vi "Phi Theta Scanning Revamped.vi"() -> ()   [LabVIEW 2022 SP3]
uses:
  C:/Users/mnopl/OneDrive/Documents/PhiThetaScanning/Thorlabs.MotionControl.Controls.dll
  Thorlabs.MotionControl.Controls.dll
  <vilib>/DAQmx/read.llb/DAQmx Read (Analog 1D DBL 1Chan NSamp).vi
  <vilib>/Analysis/baseanly.llb/Mean (DBL).vi
  <vilib>/DAQmx/miscellaneous.llb/DAQmx Fill In Error Info.vi
  C:/Users/mnopl/OneDrive/Documents/PhiThetaScanning/Thorlabs.MotionControl.KCube.StepperMotorCLI.dll
  Thorlabs.MotionControl.KCube.StepperMotorCLI.dll
  <vilib>/Analysis/NI_AALBase.lvlib
panel:
  in  "2D Flyover":bool
  in  "Flyover Y Linescan":bool
  in  "Update Vel/Acc":bool
  in  "Save Line graph":bool
  in  "Grid points":dbl=3000.0
  in  "Save Phi/Theta":bool
  out "Time Left":dbl
  out "Line Scan":dbl[](graph)
  in  "Move to Saved Pos":bool
  in  "Save Position":bool
  out "Y Pos 1":dbl
  out "X Pos 1":dbl
  out "return value":dbl[][](array[numeric])
  in  "Save Data":bool
  in  "Move to Origin":bool
  in  "Acceleration":dbl=10.0
  in  "Mesuares/Pixel":dbl=100.0
  in  "Flyover X Linescan":bool
  in  "Move Y":bool
  in  "Move X":bool
  in  "Y Step Size":dbl=1.0
  in  "X Step Size":dbl=1.0
  in  "Move to Y":bool
  in  "Move to X":bool
  in  "Y Move":dbl=1.0
  in  "X Move":dbl=1.0
  out "Y Line Scan":dbl[](array[numeric])=[-inf, -inf, -inf, -inf, -inf, -inf]
  out "X Line Scan":dbl[](array[numeric])=[-inf, -inf, -inf, -inf, -inf, -inf]
  out "Y Origin":dbl
  out "X Orign":dbl
  out "Scan Type":string="Scan"
  in  "Y Line Scan":bool
  in  "Abort":bool
  in  "X Line Scan":bool
  out "(X,Y)":cluster{dbl, dbl}[][](array[cluster])
  out "Phi Theta Data":dbl[][](graph)
  in  "Save Image":bool
  in  "Convert to phi/theta":bool
  in  "Move to Cursor":bool
  in  "Y Pos":dbl=0.899996795693412
  in  "X Pos":dbl=1.0
  in  "Read Position":bool
  out "Graph":dbl[][](graph)
  out "array of values":dbl[][](array[numeric])=[[-inf, -inf, -inf, -inf, -inf, -inf], [-inf, -inf, -inf, -inf, -inf, -inf], [-inf, -inf, -inf, -inf, -inf, -inf], [-inf, -inf, -inf, -inf, -inf, -inf], [-inf, -inf, -inf, -inf, -inf, -inf], [-inf, -inf, -inf, -inf, -inf, -inf]]
  out "task out":refnum<k21>
  in  "physical channels":tag="Dev3/ai0"
  in  "number of samples":i32=10000
  in  "rate":dbl=250000.0
  in  "maximum value":dbl=5.0 format="%0.2f"
  in  "minimum value":dbl=-5.0 format="%0.2f"
  in  "Take Single Measurement":bool
  out "Done Mov?":bool=TRUE
  in  "Y Length":dbl=5.0
  in  "X Length":dbl=5.0
  in  "2D Scan":bool
  in  "Velocity":dbl=2.0
  in  "Move Y (in)":bool
  in  "Move X (in)":bool
  in  "Time to wait":dbl=251.0
  out "Time":i32=77055304
  in  "Y Step Size (in)":dbl=1.0
  in  "X Step Size (in)":dbl=1.0
  in  "X=T,Y=F":bool
  in  "Moving?":bool
  in  "Stop":bool
  in  "KCubeStepperControl Y":refnum<k24>(container)
  in  "KCubeStepperControl X":refnum<k24>(container)
  in  "SerialNumber X":string="26005327"
  in  "SerialNumber Y":string="26005279"
  in  "Set Vel/Acc":bool
  # "Internal Variables"
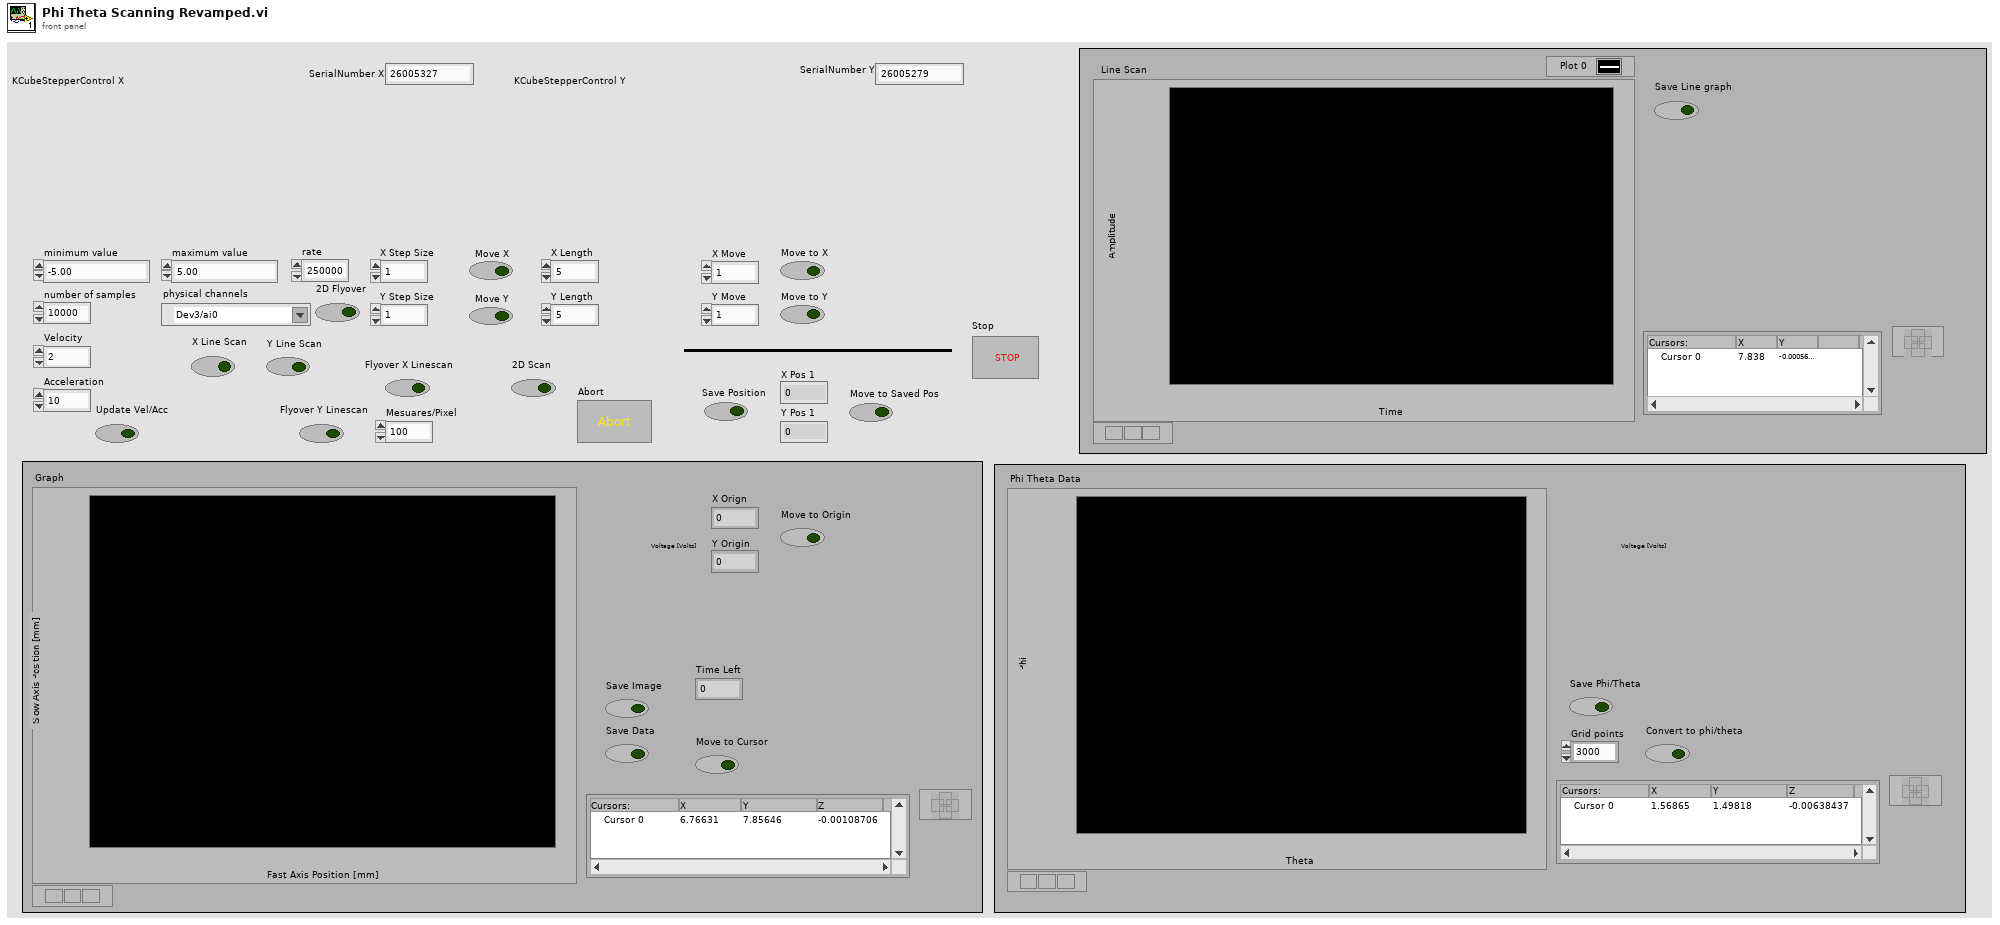
[diagram p1: front panel]
types:
  T1 = typedef "LVPointDoubleTypeDef.ctl" = cluster{"Cursor X":dbl, "Cursor Y":dbl}
  T2 = typedef "imagedata.ctl" = cluster{"image type":i32, "image depth":i32, "image":u8[], "mask":u8[], "colors":u32[], "Rectangle":cluster{"left":i16, "top":i16, "right":i16, "bottom":i16}}
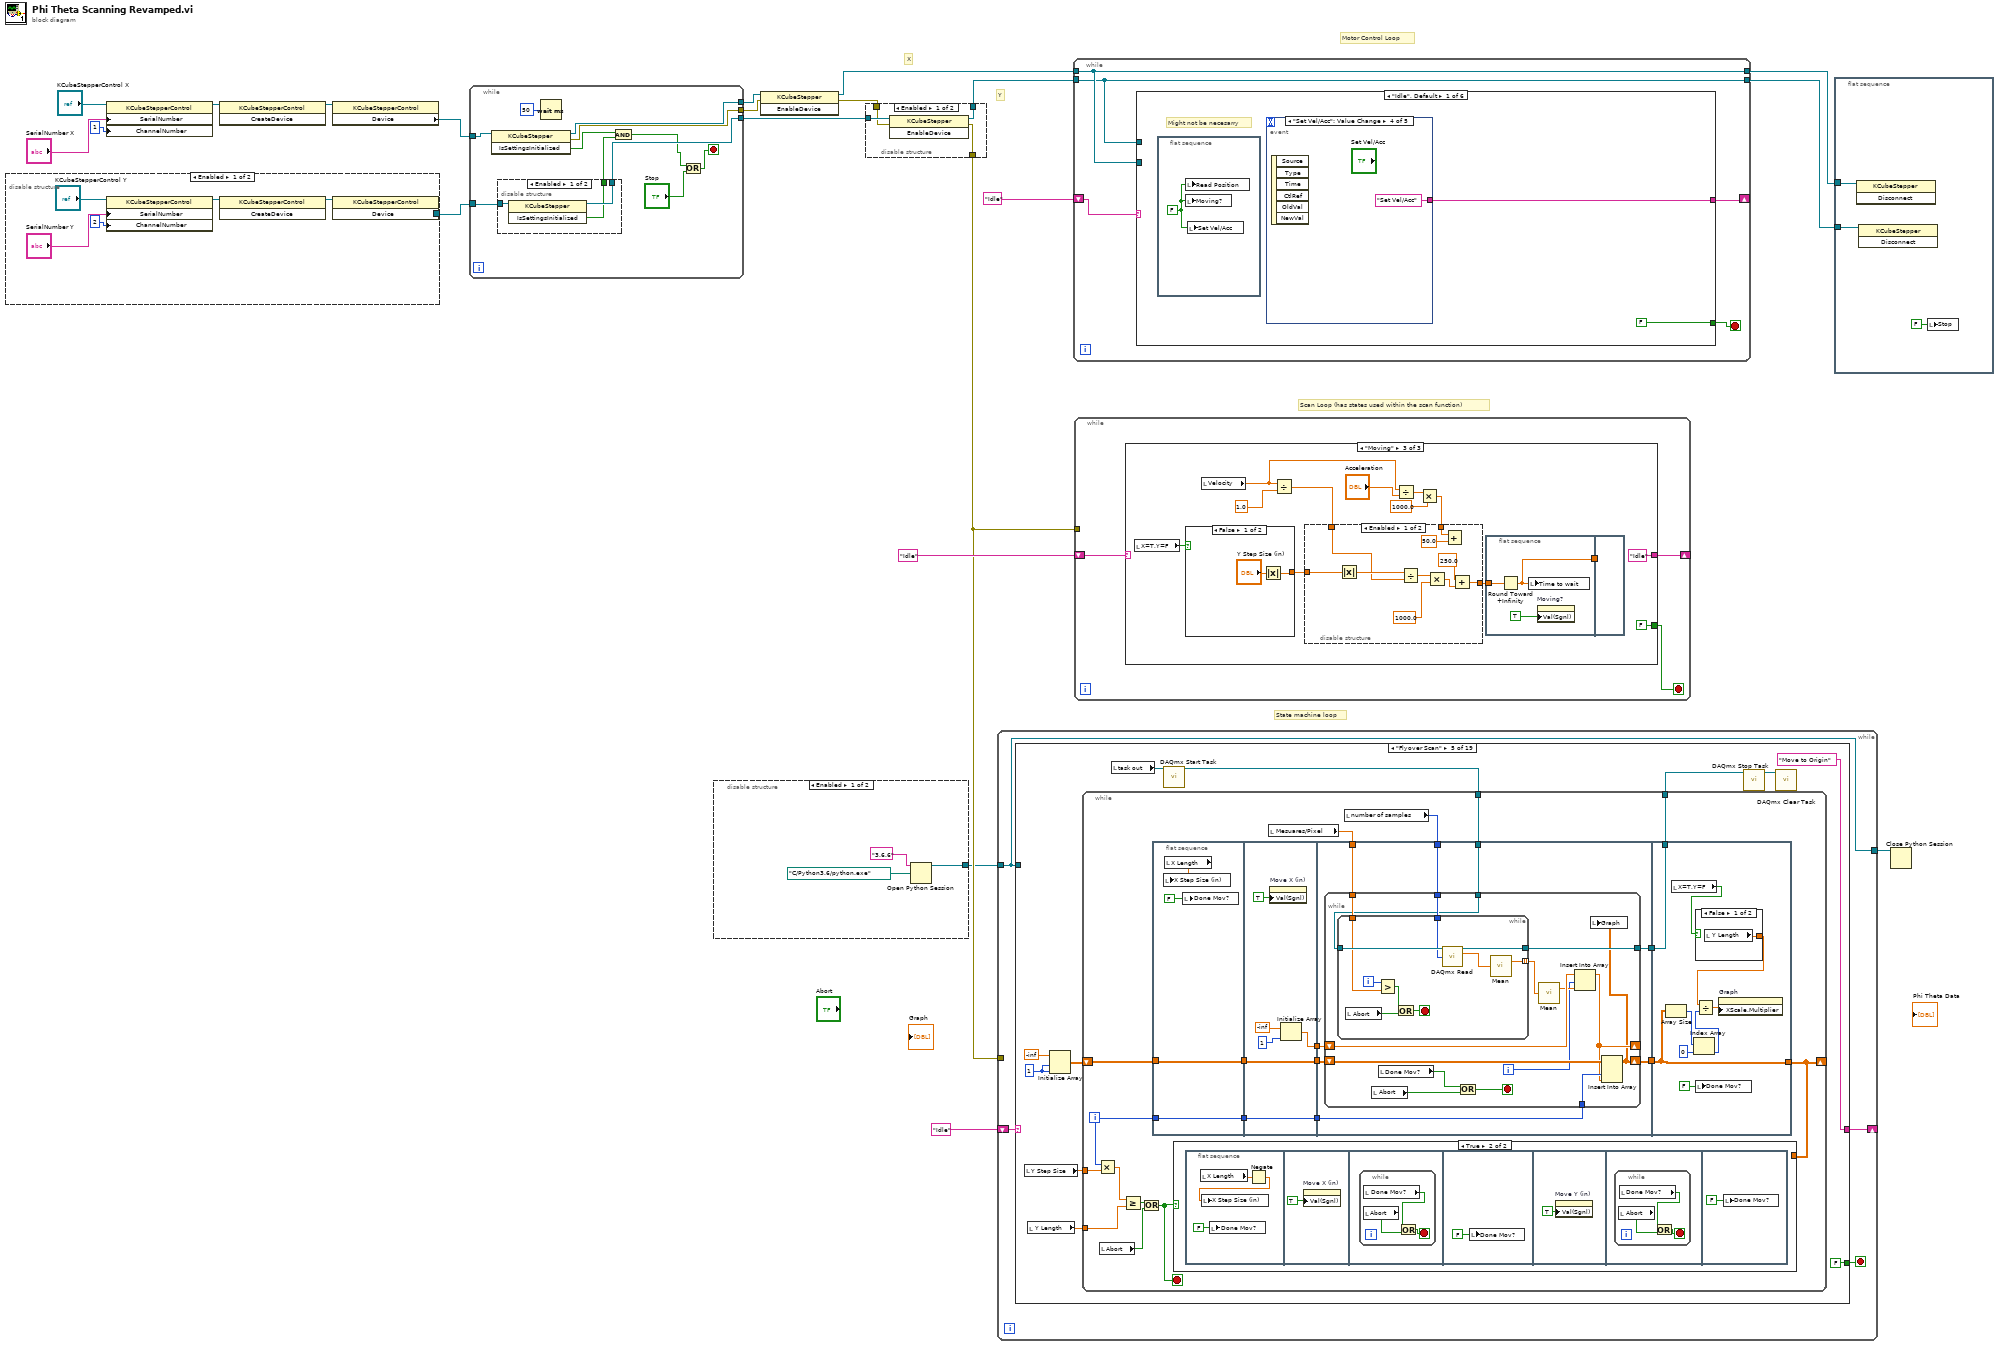
[diagram p0: block diagram]
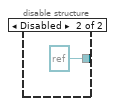
[diagram p2: hidden frame]
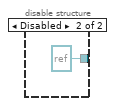
[diagram p4: hidden frame]
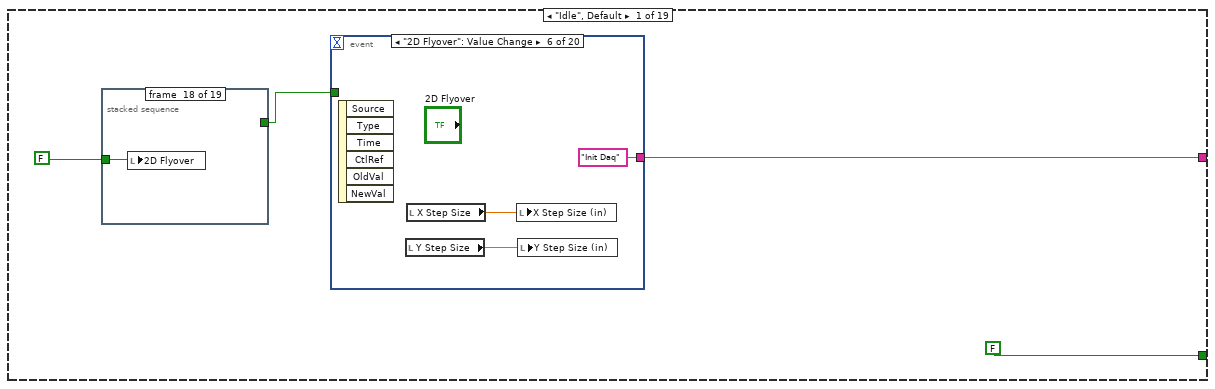
[diagram p5: hidden frame]
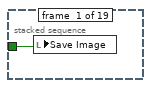
[diagram p6: hidden frame]
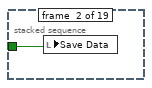
[diagram p7: hidden frame]
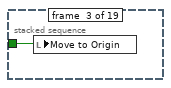
[diagram p8: hidden frame]
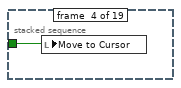
[diagram p9: hidden frame]
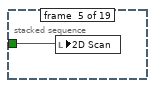
[diagram p10: hidden frame]
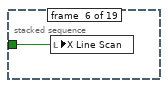
[diagram p11: hidden frame]
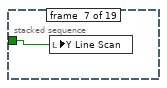
[diagram p12: hidden frame]
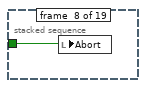
[diagram p13: hidden frame]
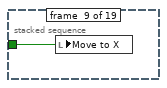
[diagram p14: hidden frame]
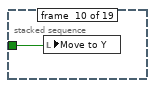
[diagram p15: hidden frame]
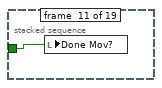
[diagram p16: hidden frame]
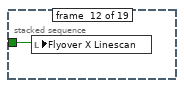
[diagram p17: hidden frame]
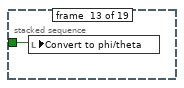
[diagram p18: hidden frame]
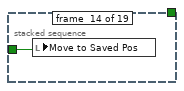
[diagram p19: hidden frame]
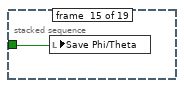
[diagram p20: hidden frame]
diagram:
  # "State machine loop"
  # "Y"
  # "X"
  # "Scan Loop (has states used within the scan function)"
  # "Motor Control Loop"
  n1 = disable-structure shown="Enabled" {
    disable-tunnel: [w23 refnum<k24> refnum ("Device")] -> w13
    frame Enabled {
      n2 = property class="KCubeStepperControl"(reference="KCubeStepperControl Y", "SerialNumber"="SerialNumber Y", "ChannelNumber"=2) -> (reference out=w26:refnum<k24>)  [unwired: 1 in, 1 out]
      n3 = invoke class="KCubeStepperControl" method="CreateDevice"(reference=w26) -> (reference out=w25:refnum<k24>)  [unwired: 2 in, 2 out]
      n4 = property class="KCubeStepperControl"(reference=w25) -> ("Device"=w23:refnum<k24>)  [unwired: 1 in, 2 out]
    }
    frame Disabled {
    }
  }
  n5 = property class="KCubeStepperControl"(reference="KCubeStepperControl X", "SerialNumber"="SerialNumber X", "ChannelNumber"=1) -> (reference out=w20:refnum<k24>)  [unwired: 1 in, 1 out]
  n6 = invoke class="KCubeStepperControl" method="CreateDevice"(reference=w20) -> (reference out=w19:refnum<k24>)  [unwired: 2 in, 2 out]
  n7 = property class="KCubeStepperControl"(reference=w19) -> ("Device"=w18:refnum<k24>)  [unwired: 1 in, 2 out]
  n8 = while {
    tunnel: w13 -> [w38]
    tunnel: w18 -> [w32]
    tunnel: [w35] -> w17
    tunnel: [w36] -> w15
    tunnel: [w37] -> w14
    stop <- w31 stop-if-true
    n9 = invoke class="KCubeStepper" method="IsSettingsInitialized"(reference=w32) -> (reference out=w36:refnum<k24>, error out=w37:errorcluster, "IsSettingsInitialized"=w33:bool)  [unwired: 2 in]
    n10 = disable-structure shown="Enabled" {
      disable-tunnel: w38 -> [w42 w43]
      disable-tunnel: [w41 w43] -> w35
      disable-tunnel: [w40 TRUE ("IsSettingsInitialized")] -> w34
      frame Enabled {
        n11 = invoke class="KCubeStepper" method="IsSettingsInitialized"(reference=w42) -> (reference out=w41:refnum<k24>, "IsSettingsInitialized"=w40:bool)  [unwired: 2 in, 1 out]
      }
      frame Disabled {
      }
    }
    n12 = Wait (ms)(milliseconds to wait=u32 50) -> ()  [unwired: 1 out]
    n13 = And(x=w33, y=w34) -> (x .and. y?=w29:bool)
    n14 = Or(x=w29, y="Stop") -> (x .or. y?=w31:bool)
  }
  n15 = disable-structure shown="Enabled" {
    disable-tunnel: [w47 refnum<k35> refnum ("session out")] -> w4
    frame Enabled {
      n16 = Open Python Session(python version="3.6.6" ("Python version"), python path=path "C:/Python3.6/python.exe" ("Python path")) -> (session out=w47:refnum<k35>)  [unwired: 1 in, 1 out]
    }
    frame Disabled {
    }
  }
  n17 = invoke class="KCubeStepper" method="EnableDevice"(reference=w15, error in=w14) -> (reference out=w2:refnum<k24>, error out=w12:errorcluster)  [unwired: 1 in, 1 out]
  n18 = disable-structure shown="Enabled" {
    disable-tunnel: w17 -> [w52 _]
    disable-tunnel: w12 -> [w51 w53]
    disable-tunnel: [w50 w53] -> w5
    disable-tunnel: [w49 _] -> w1
    frame Enabled {
      n19 = invoke class="KCubeStepper" method="EnableDevice"(reference=w52, error in=w51) -> (reference out=w49:refnum<k24>, error out=w50:errorcluster)  [unwired: 1 in, 1 out]
    }
    frame Disabled {
    }
  }
  n20 = while {
    shift-right: [w56] -> _
    shift-left: "Idle" -> [w57]
    tunnel: w5 -> [_]
    tunnel: w4 -> [w54]
    tunnel: [w54] -> w3
    stop <- w55 stop-if-true
    n21 = case shown="\"Flyover Scan\"" w57 {
      tunnel: [w61 "Init Graph" w152 "Move to Origin" "Move to Origin" ("Scan Type") "Move to Origin" ("Scan Type") "Move to Origin" ("Scan Type") "Idle" ("Scan Type") "Idle" ("Scan Type") "Idle" "Idle" ("Scan Type") "Idle" ("Scan Type") "Idle" "Idle" ("Scan Type") "Idle" "Idle" ("Scan Type") "Idle" ("Scan Type") "Idle" ("Scan Type") "Idle"] -> w56
      tunnel: [FALSE FALSE FALSE FALSE FALSE FALSE FALSE FALSE FALSE FALSE FALSE FALSE FALSE FALSE FALSE FALSE FALSE FALSE TRUE] -> w55
      tunnel: w54 -> [_ _ _ _ _ _ _ _ _ _ _ _ w791 _ _ w928 _ _ _]
      frame "Idle", Default {
        n22 = stacked-sequence {
          tunnel: FALSE -> [w62 w63 w64 w65 w66 w67 w68 w69 w70 w71 w72 w73 w74 w75 w76 w77 w78 w79 w80]
          tunnel: [_ _ _ _ _ _ _ _ _ _ _ _ _ _ _ _ _ _ w80] -> w58
          frame #0 {
            n23 = local write "Save Image"(w62) -> ()
          }
          frame #1 {
            n24 = local write "Save Data"(w63) -> ()
          }
          frame #2 {
            n25 = local write "Move to Origin"(w64) -> ()
          }
          frame #3 {
            n26 = local write "Move to Cursor"(w65) -> ()
          }
          frame #4 {
            n27 = local write "2D Scan"(w66) -> ()
          }
          frame #5 {
            n28 = local write "X Line Scan"(w67) -> ()
          }
          frame #6 {
            n29 = local write "Y Line Scan"(w68) -> ()
          }
          frame #7 {
            n30 = local write "Abort"(w69) -> ()
          }
          frame #8 {
            n31 = local write "Move to X"(w70) -> ()
          }
          frame #9 {
            n32 = local write "Move to Y"(w71) -> ()
          }
          frame #10 {
            n33 = local write "Done Mov?"(w72) -> ()
          }
          frame #11 {
            n34 = local write "Flyover X Linescan"(w73) -> ()
          }
          frame #12 {
            n35 = local write "Convert to phi/theta"(w74) -> ()
          }
          frame #13 {
            n36 = local write "Move to Saved Pos"(w75) -> ()
          }
          frame #14 {
            n37 = local write "Save Phi/Theta"(w76) -> ()
          }
          frame #15 {
            n38 = local write "Update Vel/Acc"(w77) -> ()
          }
          frame #16 {
            n39 = local write "Flyover Y Linescan"(w78) -> ()
          }
          frame #17 {
            n40 = local write "2D Flyover"(w79) -> ()
          }
          frame #18 {
            n41 = local write "Save Position"(w80) -> ()
          }
        }
        n42 = event shown="[5] \"2D Flyover\": Value Change" {
          selector: _ -> [_ _ _ _ _ _ _ _ _ _ _ _ _ _ _ _ _ _ _ _]
          dyn-events: _ -> [_ _ _ _ _ _ _ _ _ _ _ _ _ _ _ _ _ _ _ _]
          timeout: _ -> [_ _ _ _ _ _ _ _ _ _ _ _ _ _ _ _ _ _ _ _]
          tunnel: ["Idle" "Convert" "Move to Cursor" "Stop" "Init Daq" "Init Daq" "Move to Origin" "Move to Saved Position" "Init Daq" "Init Daq" "Init Daq" "Init Daq" "Move to" "Move to" "Update Vel/Acc" "Save Position" "Save Image" "Save Phi/Theta" "Save Line graph" "Save Data"] -> w61
          tunnel: w58 -> [_ _ _ _ _ _ _ _ _ _ _ _ _ _ _ _ _ _ _ _]
          event Timeout {
            n43 = event-data() -> ()  [unwired: 1 in, 3 out]
          }
          event "Convert to phi/theta": Value Change {
            n44 = event-data() -> ()  [unwired: 1 in, 6 out]
          }
          event "Move to Cursor": Value Change {
            n45 = event-data() -> ()  [unwired: 1 in, 6 out]
          }
          event "Stop": Value Change {
            n46 = event-data() -> ()  [unwired: 1 in, 6 out]
          }
          event "2D Scan": Value Change {
            n47 = event-data() -> ()  [unwired: 1 in, 6 out]
            n48 = local read "X Step Size"() -> (w85:dbl)
            n49 = local read "Y Step Size"() -> (w86:dbl)
            n50 = local write "Scan Type"("Scan" ("Scan Type")) -> ()
            n51 = local write "Y Step Size (in)"(w86) -> ()
            n52 = local write "X Step Size (in)"(w85) -> ()
          }
          event "2D Flyover": Value Change {
            n53 = event-data() -> ()  [unwired: 1 in, 6 out]
            n54 = local read "Y Step Size"() -> (w89:dbl)
            n55 = local read "X Step Size"() -> (w90:dbl)
            n56 = local write "X Step Size (in)"(w90) -> ()
            n57 = local write "Y Step Size (in)"(w89) -> ()
          }
          event "Move to Origin": Value Change {
            n58 = event-data() -> ()  [unwired: 1 in, 6 out]
          }
          event "Move to Saved Pos": Value Change {
            n59 = event-data() -> ()  [unwired: 1 in, 6 out]
          }
          event "X Line Scan": Value Change {
            n60 = event-data() -> ()  [unwired: 1 in, 6 out]
            n61 = local read "X Step Size"() -> (w94:dbl)
            n62 = local write "X Step Size (in)"(w94) -> ()
            n63 = local write "Scan Type"("Line Scan" ("Scan Type")) -> ()
            n64 = local write "X=T,Y=F"(TRUE ("X=T,Y=F")) -> ()
          }
          event "Flyover X Linescan": Value Change {
            n65 = event-data() -> ()  [unwired: 1 in, 6 out]
            n66 = local read "X Step Size"() -> (w101:dbl)
            n67 = local write "X Step Size (in)"(w101) -> ()
            n68 = local write "Scan Type"("Flyover Linescan" ("Scan Type")) -> ()
            n69 = local write "X=T,Y=F"(TRUE ("X=T,Y=F")) -> ()
          }
          event "Flyover Y Linescan": Value Change {
            n70 = event-data() -> ()  [unwired: 1 in, 6 out]
            n71 = local read "Y Step Size"() -> (w103:dbl)
            n72 = local write "Y Step Size (in)"(w103) -> ()
            n73 = local write "Scan Type"("Flyover Linescan" ("Scan Type")) -> ()
            n74 = local write "X=T,Y=F"(FALSE ("X=T,Y=F")) -> ()
          }
          event "Y Line Scan": Value Change {
            n75 = event-data() -> ()  [unwired: 1 in, 6 out]
            n76 = local read "Y Step Size"() -> (w106:dbl)
            n77 = local write "Y Step Size (in)"(w106) -> ()
            n78 = local write "X=T,Y=F"(FALSE ("X=T,Y=F")) -> ()
            "Scan Type" <- "Line Scan" ("Scan Type")
          }
          event "Move to X": Value Change {
            n79 = event-data() -> ()  [unwired: 1 in, 6 out]
            n80 = local write "X=T,Y=F"(TRUE ("X=T,Y=F")) -> ()
          }
          event "Move to Y": Value Change {
            n81 = event-data() -> ()  [unwired: 1 in, 6 out]
            n82 = local write "X=T,Y=F"(FALSE ("X=T,Y=F")) -> ()
          }
          event "Update Vel/Acc": Value Change {
            n83 = event-data() -> ()  [unwired: 1 in, 6 out]
          }
          event "Save Position": Value Change {
            n84 = event-data() -> ()  [unwired: 1 in, 6 out]
          }
          event "Save Image": Value Change {
            n85 = event-data() -> ()  [unwired: 1 in, 6 out]
          }
          event "Save Phi/Theta": Value Change {
            n86 = event-data() -> ()  [unwired: 1 in, 6 out]
          }
          event "Save Line graph": Value Change {
            n87 = event-data() -> ()  [unwired: 1 in, 6 out]
          }
          event "Save Data": Value Change {
            n88 = event-data() -> ()  [unwired: 1 in, 6 out]
          }
        }
      }
      frame "Init Daq" {
        w120 = -inf
        n89 = local read "Y Length"() -> (w133:dbl)
        n90 = local read "Y Step Size"() -> (w132:dbl)
        n91 = local read "X Length"() -> (w130:dbl)
        n92 = local read "X Step Size"() -> (w129:dbl)
        n93 = Divide(x=w133, y=w132) -> (x/y=w134:dbl)
        n94 = Divide(x=w130, y=w129) -> (x/y=w131:dbl)
        n95 = Round Toward +Infinity(x=w134) -> (ceil(x): smallest int >= x=w123:dbl)
        n96 = Round Toward +Infinity(x=w131) -> (ceil(x): smallest int >= x=w128:dbl)
        n97 = Increment(x=w123) -> (x+1=w121:dbl)
        n98 = Increment(x=w128) -> (x+1=w122:dbl)
        n99 = call "Initialize DAQ Assistant.vi"("minimum value"="minimum value", "maximum value"="maximum value", "rate"="rate", "number of samples"="number of samples", "physical channels"="physical channels") -> ("task out"=→"task out":refnum<k21>)  [unwired: 5 in, 1 out]
        n100 = Initialize Array(w120, w121) -> (→"Y Line Scan":dbl[])
        n101 = Initialize Array(w120, w122, w121) -> (→"array of values":dbl[][])
        n102 = Initialize Array(w120, w122) -> (→"X Line Scan":dbl[])
      }
      frame "Init Graph" {
        n103 = local read "Acceleration"() -> (w148:dbl)
        n104 = local read "Scan Type"() -> (w152:string)
        n105 = local read "Velocity"() -> (w149:dbl)
        n106 = flat-sequence {
          tunnel: [w205] -> w142
          tunnel: ["X Pos"] -> w154
          tunnel: ["Y Pos"] -> w153
          frame #0 {
            n107 = property on="Read Position" class="Bool (strict)"("Val(Sgnl)"=TRUE) -> ()  [unwired: 2 in, 2 out]
          }
          frame #1 {
            n108 = while {
              tunnel: [w206] -> w205
              stop <- w209 stop-if-true
              n109 = local read "Read Position"() -> (w208:bool)
              n110 = Not(x=w208) -> (.not. x?=w209:bool)
              n111 = Wait (ms)(milliseconds to wait=u32 10) -> (millisecond timer value=w206:u32)
            }
          }
          frame #2 {
            "X Orign" <- "X Pos"
            "Y Origin" <- "Y Pos"
          }
        }
        n112 = case shown="\"Scan\"" w152 {
          tunnel: [w170 w188] -> w146
          tunnel: w145 -> [w170 w188]
          frame "Line Scan", Default {
            n113 = local read "X=T,Y=F"() -> (w171:bool)
            n114 = case shown="True" w171 {
              frame False {
                n115 = flat-sequence {
                  frame #0 {
                    n116 = local read "Y Length"() -> (w173:dbl)
                    n117 = Divide(x=w173, y=2.0) -> (x/y=w174:dbl)
                    n118 = Negate(x=w174) -> (-x=w175:dbl)
                    n119 = local write "Y Step Size (in)"(w175) -> ()
                  }
                  frame #1 {
                    n120 = local write "Done Mov?"(FALSE ("Done Mov?")) -> ()
                    n121 = property on="Move Y (in)" class="Bool (strict)"("Val(Sgnl)"=TRUE ("Value (Signaling)")) -> ()  [unwired: 2 in, 2 out]
                  }
                  frame #2 {
                    n122 = while {
                      stop <- w178 stop-if-true
                      n123 = local read "Done Mov?"() -> (w178:bool)
                    }
                  }
                  frame #3 {
                    n124 = local write "Done Mov?"(FALSE ("Done Mov?")) -> ()
                  }
                }
              }
              frame True {
                n125 = flat-sequence {
                  frame #0 {
                    n126 = local read "X Length"() -> (w183:dbl)
                    n127 = Divide(x=w183, y=2.0) -> (x/y=w182:dbl)
                    n128 = Negate(x=w182) -> (-x=w181:dbl)
                    n129 = local write "X Step Size (in)"(w181) -> ()
                  }
                  frame #1 {
                    n130 = property on="Move X (in)" class="Bool (strict)"("Val(Sgnl)"=TRUE ("Value (Signaling)")) -> ()  [unwired: 2 in, 2 out]
                    n131 = local write "Done Mov?"(FALSE ("Done Mov?")) -> ()
                  }
                  frame #2 {
                    n132 = while {
                      stop <- w186 stop-if-true
                      n133 = local read "Done Mov?"() -> (w186:bool)
                    }
                  }
                  frame #3 {
                    n134 = local write "Done Mov?"(FALSE ("Done Mov?")) -> ()
                  }
                }
              }
            }
          }
          frame "Scan" {
            n135 = flat-sequence {
              frame #0 {
                n136 = local read "X Length"() -> (w196:dbl)
                n137 = local read "Y Length"() -> (w194:dbl)
                n138 = Divide(x=w196, y=2.0) -> (x/y=w192:dbl)
                n139 = Divide(x=w194, y=2.0) -> (x/y=w190:dbl)
                n140 = Negate(x=w192) -> (-x=w191:dbl)
                n141 = Negate(x=w190) -> (-x=w189:dbl)
                n142 = local write "X Step Size (in)"(w191) -> ()
                n143 = local write "Y Step Size (in)"(w189) -> ()
              }
              frame #1 {
                n144 = local write "Done Mov?"(FALSE ("Done Mov?")) -> ()
                n145 = property on="Move Y (in)" class="Bool (strict)"("Val(Sgnl)"=TRUE ("Value (Signaling)")) -> ()  [unwired: 2 in, 2 out]
              }
              frame #2 {
                n146 = while {
                  stop <- w199 stop-if-true
                  n147 = local read "Done Mov?"() -> (w199:bool)
                }
              }
              frame #3 {
                n148 = local write "Done Mov?"(FALSE ("Done Mov?")) -> ()
                n149 = property on="Move X (in)" class="Bool (strict)"("Val(Sgnl)"=TRUE ("Value (Signaling)")) -> ()  [unwired: 2 in, 2 out]
              }
              frame #4 {
                n150 = while {
                  stop <- w202 stop-if-true
                  n151 = local read "Done Mov?"() -> (w202:bool)
                }
              }
              frame #5 {
                n152 = local write "Done Mov?"(FALSE ("Done Mov?")) -> ()
              }
            }
          }
        }
        n153 = flat-sequence {
          tunnel: w149 -> [w159]
          tunnel: [w159] -> w151
          tunnel: w148 -> [w156]
          tunnel: [w156] -> w150
          tunnel: w142 -> [_]
          tunnel: w151 -> [w162]
          tunnel: w150 -> [w161]
          tunnel: [w162] -> w144
          tunnel: [w161] -> w143
          tunnel: [w164] -> w145
          tunnel: [w165] -> w147
          tunnel: w144 -> [w165]
          tunnel: w143 -> [w164]
          frame #0 {
            n154 = local write "Acceleration"(10.0 ("Acceleration")) -> ()
            n155 = local write "Velocity"(2.0 ("Velocity")) -> ()
          }
          frame #1 {
            n156 = property on="Set Vel/Acc" class="Bool (strict)"("Val(Sgnl)"=TRUE ("Value (Signaling)")) -> ()  [unwired: 2 in, 2 out]
          }
          frame #2 {
            n157 = Wait (ms)(milliseconds to wait=u32 150) -> ()  [unwired: 1 out]
          }
        }
        n158 = case shown="\"Scan\"" w152 {
          tunnel: w154 -> [w215 w234]
          tunnel: w153 -> [w214 w229]
          frame "Line Scan", Default {
            n159 = local read "X=T,Y=F"() -> (w213:bool)
            n160 = case shown="False" w213 {
              tunnel: w215 -> [_ w227]
              tunnel: w214 -> [w221 _]
              tunnel: [w216 w222] -> w212
              frame False {
                n161 = local read "Y Length"() -> (w219:dbl)
                n162 = local read "Y Step Size"() -> (w216:dbl)
                n163 = Divide(x=w219, y=2.0) -> (x/y=w217:dbl)
                n164 = Subtract(x=w221, y=w217) -> (x-y=w220:dbl)
                n165 = property on="Line Scan" class="WFGraph (strict)"("XScale.Offset"=w220) -> ()  [unwired: 2 in, 2 out]
              }
              frame True {
                n166 = local read "X Length"() -> (w225:dbl)
                n167 = Divide(x=w225, y=2.0) -> (x/y=w223:dbl)
                n168 = Subtract(x=w227, y=w223) -> (x-y=w226:dbl)
                n169 = local read "X Step Size"() -> (w222:dbl)
                n170 = property on="Line Scan" class="WFGraph (strict)"("XScale.Offset"=w226) -> ()  [unwired: 2 in, 2 out]
              }
            }
            n171 = property on="Line Scan" class="WFGraph (strict)"("XScale.Multiplier"=w212) -> ()  [unwired: 2 in, 2 out]
          }
          frame "Scan" {
            n172 = local read "X Length"() -> (w237:dbl)
            n173 = local read "Y Length"() -> (w232:dbl)
            n174 = Divide(x=w237, y=2.0) -> (x/y=w235:dbl)
            n175 = Divide(x=w232, y=2.0) -> (x/y=w230:dbl)
            n176 = local read "Y Step Size"() -> (w239:dbl)
            n177 = local read "X Step Size"() -> (w238:dbl)
            n178 = Subtract(x=w229, y=w230) -> (x-y=w228:dbl)
            n179 = Subtract(x=w234, y=w235) -> (x-y=w233:dbl)
            n180 = property on="Graph" class="IntGraph (strict)"("XScale.Offset"=w233) -> ()  [unwired: 2 in, 2 out]
            n181 = property on="Graph" class="IntGraph (strict)"("YScale.Offset"=w228) -> ()  [unwired: 2 in, 2 out]
            n182 = property on="Graph" class="IntGraph (strict)"("YScale.Multiplier"=w239) -> ()  [unwired: 2 in, 2 out]
            n183 = property on="Graph" class="IntGraph (strict)"("XScale.Multiplier"=w238) -> ()  [unwired: 2 in, 2 out]
          }
        }
        n184 = flat-sequence {
          tunnel: w146 -> [w167]
          tunnel: w147 -> [w166]
          frame #0 {
            n185 = local write "Velocity"(w166) -> ()
            n186 = local write "Acceleration"(w167) -> ()
          }
          frame #1 {
            n187 = property on="Set Vel/Acc" class="Bool (strict)"("Val(Sgnl)"=TRUE ("Value (Signaling)")) -> ()  [unwired: 2 in, 2 out]
          }
          frame #2 {
            n188 = Wait (ms)(milliseconds to wait=u32 150) -> ()  [unwired: 1 out]
          }
        }
      }
      frame "Scan" {
        w248 = 0 ("Row")
        n189 = local read "number of samples"() -> (w244:i32)
        n190 = local read "Y Step Size"() -> (w242:dbl)
        n191 = local read "array of values"() -> (w246:dbl[][])
        n192 = local read "Y Origin"() -> (w253:dbl)
        n193 = local read "task out"() -> (w247:refnum<k21>)
        n194 = local read "X Orign"() -> (w255:dbl)
        n195 = local read "X Step Size"() -> (w259:dbl)
        n196 = Divide(x="Y Length", y=2.0) -> (x/y=w251:dbl)
        n197 = Divide(x="X Length", y=2.0) -> (x/y=w254:dbl)
        n198 = Divide(x="Y Length", y=w242) -> (x/y=w241:dbl)
        n199 = call "Measure and Update Array.vi"("Array In"=w246, "number of samples per channel"=w244, "task/channels in"=w247, "Row"=w248, "Column"=w248) -> ("Array Out"=w245:dbl[][])  [unwired: 7 in, 3 out]
        n200 = local write "Graph"(w245) -> ()
        n201 = Subtract(x=w253, y=w251) -> (x-y=w249:dbl)
        n202 = Subtract(x=w255, y=w254) -> (x-y=w250:dbl)
        n203 = while {
          shift-right: [w294] -> w261
          shift-left: w245 -> [w295]
          tunnel: [w290] -> w260 mode=indexing
          tunnel: "X Length" -> [w286]
          tunnel: w259 -> [w289]
          tunnel: w242 -> [w288]
          tunnel: "Y Length" -> [w287]
          tunnel: [w280] -> w258
          tunnel: "X Length" -> [w285]
          tunnel: w250 -> [w279]
          tunnel: w249 -> [w278]
          tunnel: w241 -> [w273]
          i -> [w292]
          stop <- w297 stop-if-true
          n204 = local read "Abort"() -> (w281:bool)
          n205 = Multiply(x=w292, y=w288) -> (x*y=w291:dbl)
          n206 = while {
            tunnel: [w404] -> w284
            tunnel: w292 -> [w404]
            tunnel: [w403] -> w296
            shift-right: [w399] -> w283
            shift-left: w295 -> [w402]
            tunnel: [w401] -> w282
            tunnel: [w400] -> w293
            tunnel: w291 -> [w390]
            tunnel: [w398] -> w290 mode=indexing
            tunnel: w286 -> [w396]
            tunnel: w289 -> [w397]
            tunnel: w279 -> [w389]
            tunnel: w278 -> [w387]
            i -> [w411]
            stop <- w408 stop-if-true
            n207 = flat-sequence {
              tunnel: w397 -> [w412]
              tunnel: w396 -> [w413]
              tunnel: w411 -> [w414]
              tunnel: [w414] -> w395
              tunnel: [w413] -> w394
              tunnel: [w412] -> w393
              tunnel: [w422] -> w410
              tunnel: [w416] -> w405
              tunnel: [w421] -> w391
              tunnel: w395 -> [w417]
              tunnel: w394 -> [w419]
              tunnel: w393 -> [w418]
              tunnel: w410 -> [w424]
              tunnel: [w425] -> w409
              tunnel: [w427] -> w407
              tunnel: [w426] -> w406
              tunnel: w405 -> [w426]
              tunnel: [w438] -> w408
              tunnel: w409 -> [w438]
              tunnel: w407 -> [_]
              tunnel: w406 -> [w431]
              tunnel: w404 -> [w436]
              tunnel: [w431] -> w403
              tunnel: [w435] -> w399
              tunnel: w402 -> [w434]
              tunnel: [w433] -> w401
              tunnel: [w432] -> w400
              frame #0 {
                n208 = local write "X Step Size (in)"(w412) -> ()
              }
              frame #1 {
                n209 = Increment(x=w417) -> (x+1=w416:i32)
                n210 = local write "Done Mov?"(FALSE ("Done Moving?")) -> ()
                n211 = property on="Move X (in)" class="Bool (strict)"("Val(Sgnl)"=TRUE) -> ()  [unwired: 2 in, 2 out]
                n212 = Multiply(x=w418, y=w416) -> (x*y=w421:dbl)
                n213 = Less Or Equal?(x=w419, y=w421) -> (x <= y?=w422:bool)
              }
              frame #2 {
                n214 = while {
                  tunnel: [w429] -> w427
                  tunnel: [w428] -> w423
                  stop <- w430 stop-if-true
                  n215 = local read "Done Mov?"() -> (w429:bool)
                  n216 = local read "Abort"() -> (w428:bool)
                  n217 = Or(x=w429, y=w428) -> (x .or. y?=w430:bool)
                }
                n218 = Or(x=w424, y=w423) -> (x .or. y?=w425:bool)
              }
              frame #3 {
                n219 = local read "number of samples"() -> (w433:i32)
                n220 = local read "task out"() -> (w437:refnum<k21>)
                n221 = call "Measure and Update Array.vi"("Array In"=w434, "number of samples per channel"=w433, "task/channels in"=w437, "Row"=w431, "Column"=w436) -> ("Array Out"=w435:dbl[][], "task out"=w432:refnum<k21>)  [unwired: 7 in, 2 out]
              }
            }
            n222 = Add(x=w387, y=w390) -> (x+y=w388:dbl)
            n223 = Add(x=w391, y=w389) -> (x+y=w392:dbl)
            n224 = Bundle(w392, w388) -> (w398:cluster{dbl, dbl})  [unwired: 1 in]
            n225 = local write "Graph"(w399) -> ()
          }
          n226 = case shown="False" w281 {
            tunnel: [w311 TRUE] -> w297
            tunnel: w296 -> [w310 _]
            tunnel: [w309 w385] -> w294
            tunnel: w293 -> [w308 w384]
            tunnel: w288 -> [w307 _]
            tunnel: [w306 w384] -> w280
            tunnel: w287 -> [w305 _]
            tunnel: w285 -> [w304 _]
            tunnel: w284 -> [w303 _]
            tunnel: w283 -> [w302 w385]
            tunnel: w282 -> [w301 _]
            tunnel: [w299 w383] -> w276
            tunnel: [w298 1.0] -> w270
            frame False {
              n227 = flat-sequence {
                tunnel: w305 -> [w333]
                tunnel: w307 -> [w328]
                tunnel: w303 -> [w334]
                tunnel: [w334] -> w327
                tunnel: [w328] -> w326
                tunnel: [w333] -> w325
                tunnel: w304 -> [w332]
                tunnel: [TRUE ("Value (Signaling)")] -> w324
                tunnel: [w339] -> w323
                tunnel: [w338] -> w322
                tunnel: [w337] -> w321
                tunnel: w327 -> [w339]
                tunnel: w326 -> [w338]
                tunnel: w325 -> [w337]
                tunnel: w324 -> [w336]
                tunnel: [w335] -> w300
                tunnel: [w344] -> w320
                tunnel: [w342] -> w319
                tunnel: [w343] -> w318
                tunnel: w323 -> [w344]
                tunnel: w322 -> [w342]
                tunnel: w321 -> [w343]
                tunnel: [w341] -> w317
                tunnel: w300 -> [w340]
                tunnel: [w356] -> w316
                tunnel: [w351] -> w315
                tunnel: w320 -> [w352]
                tunnel: w319 -> [w354]
                tunnel: w318 -> [w349]
                tunnel: w317 -> [_]
                tunnel: [w348] -> w298
                tunnel: w316 -> [w359]
                tunnel: [w357] -> w314
                tunnel: [w361] -> w313
                tunnel: [w360] -> w312
                tunnel: w315 -> [w360]
                tunnel: [w366] -> w311
                tunnel: w314 -> [w366]
                tunnel: w313 -> [_]
                tunnel: w312 -> [w372]
                tunnel: w310 -> [_]
                tunnel: [w368] -> w309
                tunnel: w302 -> [w371]
                tunnel: w301 -> [w370]
                tunnel: w308 -> [w369]
                tunnel: [w367] -> w306
                tunnel: [w365] -> w299
                frame #0 {
                  n228 = Negate(x=w332) -> (-x=w330:dbl)
                  n229 = local write "X Step Size (in)"(w330) -> ()
                  n230 = local write "Y Step Size (in)"(w328) -> ()
                  n231 = local write "Done Mov?"(FALSE ("Done Moving?")) -> ()
                }
                frame #1 {
                  n232 = property on="Move X (in)" class="Bool (strict)"("Val(Sgnl)"=w336) -> (error out=w335:errorcluster)  [unwired: 2 in, 1 out]
                }
                frame #2 {
                  n233 = while {
                    tunnel: [w345] -> w341
                    tunnel: w340 -> [_]
                    stop <- w347 stop-if-true
                    n234 = local read "Done Mov?"() -> (w345:bool)
                    n235 = local read "Abort"() -> (w346:bool)
                    n236 = Or(x=w346, y=w345) -> (x .or. y?=w347:bool)
                  }
                }
                frame #3 {
                  n237 = local write "Done Mov?"(FALSE ("Done Mov?")) -> ()
                  n238 = property on="Move Y (in)" class="Bool (strict)"("Val(Sgnl)"=TRUE) -> ()  [unwired: 2 in, 2 out]
                  n239 = Multiply(x=w354, y=w352) -> (x*y=w350:dbl)
                  n240 = Increment(x=w352) -> (x+1=w351:i32)
                  n241 = Divide(x=w350, y=w349) -> (x/y=w348:dbl)
                  n242 = Less Or Equal?(x=w349, y=w350) -> (x <= y?=w356:bool)
                }
                frame #4 {
                  n243 = while {
                    tunnel: [w363] -> w361
                    tunnel: [w362] -> w358
                    stop <- w364 stop-if-true
                    n244 = local read "Done Mov?"() -> (w363:bool)
                    n245 = local read "Abort"() -> (w362:bool)
                    n246 = Or(x=w363, y=w362) -> (x .or. y?=w364:bool)
                  }
                  n247 = Or(x=w359, y=w358) -> (x .or. y?=w357:bool)
                }
                frame #5 {
                  n248 = case shown="False" w366 {
                    tunnel: w372 -> [w379 _]
                    tunnel: w371 -> [w378 w381]
                    tunnel: w370 -> [w377 _]
                    tunnel: w369 -> [w376 w380]
                    tunnel: [w375 w381] -> w368
                    tunnel: [w374 w380] -> w367
                    frame False {
                      n249 = call "Measure and Update Array.vi"("Array In"=w378, "number of samples per channel"=w377, "task/channels in"=w376, "Row"=0, "Column"=w379) -> ("Array Out"=w375:dbl[][], "task out"=w374:refnum<k21>)  [unwired: 7 in, 2 out]
                      n250 = local write "Graph"(w375) -> ()
                    }
                    frame True {
                    }
                  }
                  n251 = Tick Count (ms)() -> (millisecond timer value=w365:u32)
                }
              }
            }
            frame True {
              n252 = Tick Count (ms)() -> (millisecond timer value=w383:u32)
            }
          }
          n253 = Tick Count (ms)() -> (millisecond timer value=w277:u32)
          n254 = Subtract(x=1.0, y=w270) -> (x-y=w272:dbl)
          n255 = Subtract(x=w276, y=w277) -> (x-y=w275:u32)
          n256 = Multiply(x=w275, y=w272) -> (x*y=w274:dbl)
          n257 = Multiply(x=w274, y=w273) -> (x*y=w267:dbl)
          n258 = Divide(x=w267, y=60000.0) -> (x/y=→"Time Left":dbl)
        }
        n259 = local write "array of values"(w261) -> ()
        n260 = flat-sequence {
          tunnel: w260 -> [w266]
          tunnel: w240 -> [w264]
          frame #0 {
            n261 = local write "Done Mov?"(FALSE) -> ()
            n262 = Wait (ms)(milliseconds to wait=w264) -> ()  [unwired: 1 out]
            "(X,Y)" <- w266
          }
        }
        n263 = local read "Time to wait"() -> (w240:dbl)
        n264 = call <vilib>:"DAQmx Clear Task.vi"("task in"=w258) -> ()  [unwired: 14 in, 1 out]
      }
      frame "Flyover Scan" {
        w446 = 1 ("dimension size")
        n265 = local read "Y Step Size"() -> (w440:dbl)
        n266 = local read "Y Length"() -> (w439:dbl)
        n267 = Initialize Array(-inf, w446, w446) -> (w445:dbl[][])
        n268 = local read "task out"() -> (w444:refnum<k21>)
        n269 = call <vilib>:"DAQmx Start Task.vi"("task/channels in"=w444) -> ("task out"=w443:refnum<k21>)  [unwired: 13 in, 1 out]
        n270 = while {
          shift-right: [w457] -> _
          shift-left: w445 -> [w463]
          tunnel: w443 -> [w459]
          tunnel: [w458] -> w442
          tunnel: w440 -> [w455]
          tunnel: w439 -> [w453]
          i -> [w456]
          stop <- w450 stop-if-true
          n271 = Multiply(x=w456, y=w455) -> (x*y=w454:dbl)
          n272 = local read "Abort"() -> (w451:bool)
          n273 = Greater Or Equal?(x=w454, y=w453) -> (x >= y?=w452:bool)
          n274 = Or(x=w452, y=w451) -> (x .or. y?=w450:bool)
          n275 = flat-sequence {
            tunnel: [w484] -> w464
            tunnel: w463 -> [w484]
            tunnel: [w483] -> w461
            tunnel: w456 -> [w483]
            tunnel: [w492] -> w465
            tunnel: w464 -> [w492]
            tunnel: [w490] -> w462
            tunnel: w461 -> [w490]
            tunnel: [w487] -> w460
            tunnel: w467 -> [w500]
            tunnel: w466 -> [w498]
            tunnel: [w499] -> w469
            tunnel: [w497] -> w468
            tunnel: w465 -> [w496]
            tunnel: w462 -> [w495]
            tunnel: w460 -> [w494]
            tunnel: w459 -> [w493]
            tunnel: w469 -> [w527]
            tunnel: w468 -> [w526]
            tunnel: [w527] -> w458
            tunnel: [w526] -> w457
            frame #0 {
              n276 = local read "X Length"() -> (w485:dbl)
              n277 = local write "X Step Size (in)"(w485) -> ()
              n278 = local write "Done Mov?"(FALSE ("Done Moving?")) -> ()
            }
            frame #1 {
              n279 = property on="Move X (in)" class="Bool (strict)"("Val(Sgnl)"=TRUE ("Value (Signaling)")) -> ()  [unwired: 2 in, 2 out]
              n280 = Initialize Array(-inf, 1 ("dimension size")) -> (w487:dbl[])
            }
            frame #2 {
              n281 = while {
                tunnel: w500 -> [w515]
                tunnel: [w514] -> w499
                tunnel: w498 -> [w510]
                shift-right: [w502] -> w497
                shift-left: w496 -> [w509]
                tunnel: w495 -> [w507]
                shift-right: [w504] -> _
                shift-left: w494 -> [w506]
                tunnel: w493 -> [w501]
                i -> [w503]
                stop <- w511 stop-if-true
                n282 = while {
                  tunnel: w515 -> [w520]
                  tunnel: w501 -> [w523]
                  tunnel: [w522] -> w514
                  tunnel: w510 -> [w517]
                  tunnel: [w516] -> w508 mode=indexing
                  i -> [w519]
                  stop <- w525 stop-if-true
                  n283 = local read "Abort"() -> (w524:bool)
                  n284 = Greater?(x=w519, y=w517) -> (0:w518:bool)
                  n285 = Or(x=w518, y=w524) -> (x .or. y?=w525:bool)
                  n286 = call-poly <vilib>:"DAQmx Read.vi"("task/channels in"=w523, "number of samples per channel"=w520) -> ("task out"=w522:refnum<k21>, "data"=w521:dbl[])  [unwired: 11 in, 1 out]
                  n287 = call-poly <vilib>:"Mean.vi"("X"=w521) -> ("mean"=w516:dbl)  [unwired: 1 out]
                }
                n288 = local read "Abort"() -> (w513:bool)
                n289 = local read "Done Mov?"() -> (w512:bool)
                n290 = Or(x=w512, y=w513) -> (x .or. y?=w511:bool)
                n291 = call-poly <vilib>:"Mean.vi"("X"=w508) -> ("mean"=w505:dbl)  [unwired: 1 out]
                n292 = Insert Into Array(array=w506, index=w503, new element=w505) -> (w504:dbl[])
                n293 = Insert Into Array(array=w509, index (col)=w507, new element=w504) -> (w502:dbl[][])  [unwired: 1 in]
                n294 = local write "Graph"(w502) -> ()
              }
            }
            frame #3 {
              n295 = Array Size(array=w526) -> (size(s)=w531:i32[])
              n296 = local read "X=T,Y=F"() -> (w533:bool)
              n297 = Index Array(array=w531, index=0) -> (element=w528:i32)
              n298 = case shown="False" w533 {
                tunnel: [w535 w536] -> w532
                frame False {
                  n299 = local read "Y Length"() -> (w535:dbl)
                }
                frame True {
                  n300 = local read "X Length"() -> (w536:dbl)
                }
              }
              n301 = Divide(x=w532, y=w528) -> (x/y=w529:dbl)
              n302 = local write "Done Mov?"(FALSE ("Done Mov?")) -> ()
              n303 = property on="Graph" class="IntGraph (strict)"("XScale.Multiplier"=w529) -> ()  [unwired: 2 in, 2 out]
            }
          }
          n304 = case shown="True" w450 {
            tunnel: w457 -> [_ _]
            frame False {
            }
            frame True {
              n305 = flat-sequence {
                frame #0 {
                  n306 = local read "X Length"() -> (w472:dbl)
                  n307 = local write "Done Mov?"(FALSE ("Done Mov?")) -> ()
                  n308 = Negate(x=w472) -> (-x=w471:dbl)
                  n309 = local write "X Step Size (in)"(w471) -> ()
                }
                frame #1 {
                  n310 = property on="Move X (in)" class="Bool (strict)"("Val(Sgnl)"=TRUE ("Value (Signaling)")) -> ()  [unwired: 2 in, 2 out]
                }
                frame #2 {
                  n311 = while {
                    stop <- w476 stop-if-true
                    n312 = local read "Abort"() -> (w474:bool)
                    n313 = local read "Done Mov?"() -> (w475:bool)
                    n314 = Or(x=w475, y=w474) -> (x .or. y?=w476:bool)
                  }
                }
                frame #3 {
                  n315 = local write "Done Mov?"(FALSE ("Done Mov?")) -> ()
                }
                frame #4 {
                  n316 = property on="Move Y (in)" class="Bool (strict)"("Val(Sgnl)"=TRUE ("Value (Signaling)")) -> ()  [unwired: 2 in, 2 out]
                }
                frame #5 {
                  n317 = while {
                    stop <- w481 stop-if-true
                    n318 = local read "Abort"() -> (w479:bool)
                    n319 = local read "Done Mov?"() -> (w480:bool)
                    n320 = Or(x=w480, y=w479) -> (x .or. y?=w481:bool)
                  }
                }
                frame #6 {
                  n321 = local write "Done Mov?"(FALSE ("Done Mov?")) -> ()
                }
              }
            }
          }
          n322 = local read "Mesuares/Pixel"() -> (w466:dbl)
          n323 = local read "number of samples"() -> (w467:i32)
        }
        n324 = call <vilib>:"DAQmx Stop Task.vi"("task/channels in"=w442) -> ("task out"=w441:refnum<k21>)  [unwired: 13 in, 1 out]
        n325 = call <vilib>:"DAQmx Clear Task.vi"("task in"=w441) -> ()  [unwired: 14 in, 1 out]
      }
      frame "Line Scan" {
        n326 = local read "X=T,Y=F"() -> (w541:bool)
        n327 = local read "X Step Size"() -> (w537:dbl)
        n328 = case shown="False" w541 {
          tunnel: [w545 w546] -> w540
          frame False {
            n329 = local read "Y Step Size"() -> (w544:dbl)
            n330 = local read "Y Line Scan"() -> (w545:dbl[])
            n331 = local write "Y Step Size (in)"(w544) -> ()
          }
          frame True {
            n332 = local read "X Line Scan"() -> (w546:dbl[])
          }
        }
        n333 = local read "X Length"() -> (w539:dbl)
        n334 = local write "X Step Size (in)"(w537) -> ()
        n335 = while {
          tunnel: w541 -> [w560]
          shift-right: [w552] -> _
          shift-left: w540 -> [w553]
          tunnel: w539 -> [w549]
          tunnel: w537 -> [w548]
          tunnel: [w547] -> w538
          i -> [w559]
          stop <- w556 stop-if-true
          n336 = flat-sequence {
            tunnel: w560 -> [w566]
            tunnel: w559 -> [w563]
            tunnel: [w565] -> w558
            tunnel: [w564] -> w554
            tunnel: w553 -> [w564]
            tunnel: [w563] -> w550
            tunnel: w549 -> [w562]
            tunnel: w548 -> [w561]
            tunnel: w558 -> [w584]
            tunnel: [w583] -> w557
            tunnel: [w582] -> w555
            tunnel: w554 -> [w582]
            tunnel: [w581] -> w551
            tunnel: w550 -> [w581]
            tunnel: [w595] -> w556
            tunnel: w557 -> [w595]
            tunnel: w555 -> [w592]
            tunnel: [w591] -> w552
            tunnel: w551 -> [w590]
            tunnel: [w588] -> w547
            frame #0 {
              n337 = case shown="False" w566 {
                tunnel: w563 -> [w571 w576]
                tunnel: [w568 w577] -> w565
                tunnel: w562 -> [_ w575]
                tunnel: w561 -> [_ w574]
                frame False {
                  n338 = local read "Y Step Size (in)"() -> (w567:dbl)
                  n339 = local read "Y Length"() -> (w569:dbl)
                  n340 = Increment(x=w571) -> (x+1=w572:i32)
                  n341 = property on="Move Y (in)" class="Bool (strict)"("Val(Sgnl)"=TRUE ("Value (Signaling)")) -> ()  [unwired: 2 in, 2 out]
                  n342 = Multiply(x=w572, y=w567) -> (x*y=w570:dbl)
                  n343 = Less Or Equal?(x=w569, y=w570) -> (x <= y?=w568:bool)
                }
                frame True {
                  n344 = property on="Move X (in)" class="Bool (strict)"("Val(Sgnl)"=TRUE ("Value (Signaling)")) -> ()  [unwired: 2 in, 2 out]
                  n345 = Multiply(x=w576, y=w574) -> (x*y=w578:dbl)
                  n346 = Less Or Equal?(x=w575, y=w578) -> (x <= y?=w577:bool)
                }
              }
            }
            frame #1 {
              n347 = while {
                tunnel: [w585] -> w580
                stop <- w587 stop-if-true
                n348 = local read "Abort"() -> (w585:bool)
                n349 = local read "Done Mov?"() -> (w586:bool)
                n350 = Or(x=w586, y=w585) -> (x .or. y?=w587:bool)
              }
              n351 = Or(x=w584, y=w580) -> (x .or. y?=w583:bool)
            }
            frame #2 {
              n352 = local read "number of samples"() -> (w593:i32)
              n353 = local read "task out"() -> (w594:refnum<k21>)
              n354 = local write "Done Mov?"(FALSE ("Done Moving?")) -> ()
              n355 = call "Measure Line Scan.vi"("number of samples per channel"=w593, "Iterator"=w590, "task/channels in"=w594, "Array in"=w592) -> ("task out"=w588:refnum<k21>, "Array out"=w591:dbl[])  [unwired: 4 in, 2 out]
            }
          }
          "Line Scan" <- w552
        }
        n356 = call <vilib>:"DAQmx Clear Task.vi"("task in"=w538) -> ()  [unwired: 14 in, 1 out]
      }
      frame "Flyover Linescan" {
        n357 = flat-sequence {
          tunnel: [w608] -> w600
          tunnel: [w613] -> w601
          tunnel: w600 -> [w614]
          tunnel: [w610] -> w598
          tunnel: w602 -> [w622]
          tunnel: w601 -> [w621]
          tunnel: "Mesuares/Pixel" -> [w619]
          tunnel: w598 -> [w618]
          tunnel: [w620] -> w597
          tunnel: [w617] -> w596
          tunnel: w597 -> [w651]
          tunnel: w596 -> [w649]
          frame #0 {
            n358 = local read "X Length"() -> (w607:dbl)
            n359 = local read "Y Length"() -> (w605:dbl)
            n360 = local write "Done Mov?"(FALSE ("Done Moving?")) -> ()
            n361 = local write "X Step Size (in)"(w607) -> ()
            n362 = local write "Y Step Size (in)"(w605) -> ()
            n363 = local read "task out"() -> (w608:refnum<k21>)
          }
          frame #1 {
            n364 = local read "X=T,Y=F"() -> (w612:bool)
            n365 = call <vilib>:"DAQmx Start Task.vi"("task/channels in"=w614) -> ("task out"=w613:refnum<k21>)  [unwired: 13 in, 1 out]
            n366 = case shown="False" w612 {
              frame False {
                n367 = property on="Move Y (in)" class="Bool (strict)"("Val(Sgnl)"=TRUE ("Value (Signaling)")) -> ()  [unwired: 2 in, 2 out]
              }
              frame True {
                n368 = property on="Move X (in)" class="Bool (strict)"("Val(Sgnl)"=TRUE ("Value (Signaling)")) -> ()  [unwired: 2 in, 2 out]
              }
            }
            n369 = Initialize Array(-inf, 1 ("dimension size")) -> (w610:dbl[])
          }
          frame #2 {
            n370 = while {
              tunnel: w622 -> [w634]
              tunnel: w621 -> [w633]
              tunnel: [w632] -> w620
              tunnel: w619 -> [w628]
              shift-right: [w625] -> w617
              shift-left: w618 -> [w627]
              i -> [w626]
              stop <- w629 stop-if-true
              n371 = while {
                tunnel: w634 -> [w639]
                tunnel: w633 -> [w642]
                tunnel: [w641] -> w632
                tunnel: w628 -> [w636]
                tunnel: [w635] -> w624 mode=indexing
                i -> [w638]
                stop <- w644 stop-if-true
                n372 = local read "Abort"() -> (w643:bool)
                n373 = Greater?(x=w638, y=w636) -> (0:w637:bool)
                n374 = Or(x=w637, y=w643) -> (x .or. y?=w644:bool)
                n375 = call-poly <vilib>:"DAQmx Read.vi"("task/channels in"=w642, "number of samples per channel"=w639) -> ("task out"=w641:refnum<k21>, "data"=w640:dbl[])  [unwired: 11 in, 1 out]
                n376 = call-poly <vilib>:"Mean.vi"("X"=w640) -> ("mean"=w635:dbl)  [unwired: 1 out]
              }
              n377 = local read "Abort"() -> (w631:bool)
              n378 = local read "Done Mov?"() -> (w630:bool)
              n379 = Or(x=w630, y=w631) -> (x .or. y?=w629:bool)
              n380 = call-poly <vilib>:"Mean.vi"("X"=w624) -> ("mean"=w623:dbl)  [unwired: 1 out]
              n381 = Insert Into Array(array=w627, index=w626, new element=w623) -> (w625:dbl[])
              n382 = local write "Line Scan"(w625) -> ()
            }
          }
          frame #3 {
            n383 = Array Size(array=w649) -> (size(s)=w648:i32)
            n384 = local read "X=T,Y=F"() -> (w646:bool)
            n385 = call <vilib>:"DAQmx Stop Task.vi"("task/channels in"=w651) -> ("task out"=w652:refnum<k21>)  [unwired: 13 in, 1 out]
            n386 = local write "Done Mov?"(FALSE ("Done Mov?")) -> ()
            n387 = case shown="False" w646 {
              tunnel: [w653 w654] -> w645
              frame False {
                n388 = local read "Y Length"() -> (w653:dbl)
              }
              frame True {
                n389 = local read "X Length"() -> (w654:dbl)
              }
            }
            n390 = Divide(x=w645, y=w648) -> (x/y=w647:dbl)
            n391 = call <vilib>:"DAQmx Clear Task.vi"("task in"=w652) -> ()  [unwired: 14 in, 1 out]
            n392 = property on="Line Scan" class="WFGraph (strict)"("XScale.Multiplier"=w647) -> ()  [unwired: 2 in, 2 out]
          }
        }
        n393 = local read "number of samples"() -> (w602:i32)
      }
      frame "Move to Origin" {
        n394 = local read "Acceleration"() -> (w663:dbl)
        n395 = local read "Velocity"() -> (w664:dbl)
        n396 = flat-sequence {
          tunnel: w665 -> [_]
          tunnel: w657 -> [w681]
          tunnel: w656 -> [w680]
          frame #0 {
            n397 = while {
              stop <- w679 stop-if-true
              n398 = local read "Done Mov?"() -> (w679:bool)
              n399 = Wait (ms)(milliseconds to wait=u32 10) -> ()  [unwired: 1 out]
            }
          }
          frame #1 {
            n400 = local write "Done Mov?"(FALSE ("Done Mov?")) -> ()
            n401 = local write "Acceleration"(w680) -> ()
            n402 = local write "Velocity"(w681) -> ()
          }
          frame #2 {
            n403 = property on="Set Vel/Acc" class="Bool (strict)"("Val(Sgnl)"=TRUE ("Value (Signaling)")) -> ()  [unwired: 2 in, 2 out]
          }
          frame #3 {
            n404 = Wait (ms)(milliseconds to wait=u32 150) -> ()  [unwired: 1 out]
          }
        }
        n405 = flat-sequence {
          tunnel: w658 -> [w686]
          tunnel: [w686] -> w657
          tunnel: [w685] -> w656
          tunnel: w655 -> [w685]
          tunnel: [w701] -> w665
          frame #0 {
            n406 = property on="Read Position" class="Bool (strict)"("Val(Sgnl)"=TRUE ("Value (Signaling)")) -> ()  [unwired: 2 in, 2 out]
            n407 = Wait (ms)(milliseconds to wait=u32 120) -> ()  [unwired: 1 out]
          }
          frame #1 {
            n408 = while {
              stop <- w689 stop-if-true
              n409 = local read "Read Position"() -> (w690:bool)
              n410 = Wait (ms)(milliseconds to wait=u32 10) -> ()  [unwired: 1 out]
              n411 = Not(x=w690) -> (.not. x?=w689:bool)
            }
          }
          frame #2 {
            n412 = local read "Y Origin"() -> (w696:dbl)
            n413 = local read "X Orign"() -> (w693:dbl)
            n414 = local read "Y Pos"() -> (w695:dbl)
            n415 = local read "X Pos"() -> (w692:dbl)
            n416 = Subtract(x=w696, y=w695) -> (x-y=w697:dbl)
            n417 = Subtract(x=w693, y=w692) -> (x-y=w694:dbl)
            n418 = local write "Y Step Size (in)"(w697) -> ()
            n419 = local write "X Step Size (in)"(w694) -> ()
          }
          frame #3 {
            n420 = local write "Done Mov?"(FALSE ("Done Mov?")) -> ()
            n421 = property on="Move X (in)" class="Bool (strict)"("Val(Sgnl)"=TRUE ("Value (Signaling)")) -> ()  [unwired: 2 in, 2 out]
          }
          frame #4 {
            n422 = while {
              stop <- w700 stop-if-true
              n423 = local read "Done Mov?"() -> (w700:bool)
            }
          }
          frame #5 {
            n424 = local write "Done Mov?"(FALSE ("Done Mov?")) -> ()
            n425 = property on="Move Y (in)" class="Bool (strict)"("Val(Sgnl)"=TRUE ("Value (Signaling)")) -> (error out=w701:errorcluster)  [unwired: 2 in, 1 out]
          }
        }
        n426 = flat-sequence {
          tunnel: w664 -> [w668]
          tunnel: w663 -> [w669]
          tunnel: [w669] -> w661
          tunnel: [w668] -> w659
          tunnel: [w673] -> w662
          tunnel: w661 -> [w673]
          tunnel: [w672] -> w660
          tunnel: w659 -> [w672]
          tunnel: [w676] -> w655
          tunnel: w662 -> [w676]
          tunnel: w660 -> [w675]
          tunnel: [w675] -> w658
          frame #0 {
            n427 = local write "Acceleration"(10.0 ("Acceleration")) -> ()
            n428 = local write "Velocity"(2.0 ("Velocity")) -> ()
          }
          frame #1 {
            n429 = property on="Set Vel/Acc" class="Bool (strict)"("Val(Sgnl)"=TRUE ("Value (Signaling)")) -> ()  [unwired: 2 in, 2 out]
          }
          frame #2 {
            n430 = Wait (ms)(milliseconds to wait=u32 150) -> ()  [unwired: 1 out]
          }
        }
      }
      frame "Move to Saved Position" {
        n431 = flat-sequence {
          tunnel: [w724] -> w704
          frame #0 {
            n432 = property on="Read Position" class="Bool (strict)"("Val(Sgnl)"=TRUE ("Value (Signaling)")) -> ()  [unwired: 2 in, 2 out]
            n433 = Wait (ms)(milliseconds to wait=u32 120) -> ()  [unwired: 1 out]
          }
          frame #1 {
            n434 = while {
              stop <- w712 stop-if-true
              n435 = local read "Read Position"() -> (w713:bool)
              n436 = Wait (ms)(milliseconds to wait=u32 10) -> ()  [unwired: 1 out]
              n437 = Not(x=w713) -> (.not. x?=w712:bool)
            }
          }
          frame #2 {
            n438 = local read "X Pos 1"() -> (w719:dbl)
            n439 = local read "Y Pos 1"() -> (w717:dbl)
            n440 = local read "X Pos"() -> (w720:dbl)
            n441 = local read "Y Pos"() -> (w716:dbl)
            n442 = Subtract(x=w719, y=w720) -> (x-y=w718:dbl)
            n443 = Subtract(x=w717, y=w716) -> (x-y=w715:dbl)
            n444 = local write "Y Step Size (in)"(w715) -> ()
            n445 = local write "X Step Size (in)"(w718) -> ()
          }
          frame #3 {
            n446 = local write "Done Mov?"(FALSE ("Done Mov?")) -> ()
            n447 = property on="Move X (in)" class="Bool (strict)"("Val(Sgnl)"=TRUE ("Value (Signaling)")) -> ()  [unwired: 2 in, 2 out]
          }
          frame #4 {
            n448 = while {
              stop <- w723 stop-if-true
              n449 = local read "Done Mov?"() -> (w723:bool)
            }
          }
          frame #5 {
            n450 = local write "Done Mov?"(FALSE ("Done Mov?")) -> ()
            n451 = property on="Move Y (in)" class="Bool (strict)"("Val(Sgnl)"=TRUE ("Value (Signaling)")) -> (error out=w724:errorcluster)  [unwired: 2 in, 1 out]
          }
        }
        n452 = flat-sequence {
          tunnel: w704 -> [_]
          frame #0 {
            n453 = while {
              stop <- w708 stop-if-true
              n454 = local read "Done Mov?"() -> (w708:bool)
              n455 = Wait (ms)(milliseconds to wait=u32 10) -> ()  [unwired: 1 out]
            }
          }
          frame #1 {
            n456 = local write "Done Mov?"(FALSE ("Done Mov?")) -> ()
          }
        }
      }
      frame "Move to Cursor" {
        n457 = flat-sequence {
          tunnel: w729 -> [_]
          tunnel: [w742] -> w733
          tunnel: w733 -> [w752]
          tunnel: [w753] -> w727
          tunnel: [w755] -> w728
          tunnel: w727 -> [w755]
          frame #0 {
            n458 = while {
              stop <- w740 stop-if-true
              n459 = local read "Read Position"() -> (w741:bool)
              n460 = Not(x=w741) -> (.not. x?=w740:bool)
              n461 = Wait (ms)(milliseconds to wait=u32 10) -> ()  [unwired: 1 out]
            }
          }
          frame #1 {
            n462 = property on="Graph" class="IntGraph (strict)"("Active Cursor"=u32 0) -> (error out=w743:errorcluster)  [unwired: 2 in, 1 out]
            n463 = property on="Graph" class="IntGraph (strict)"(error in=w743) -> ("Cursor.Cursor Position"=w742:T1)  [unwired: 1 in, 2 out]
          }
          frame #2 {
            n464 = Unbundle By Name(w752) -> ("Cursor X"=w751:dbl, "Cursor Y"=w746:dbl)
            n465 = local read "X Pos"() -> (w750:dbl)
            n466 = local read "Y Pos"() -> (w749:dbl)
            n467 = Subtract(x=w751, y=w750) -> (x-y=w748:dbl)
            n468 = Subtract(x=w746, y=w749) -> (x-y=w747:dbl)
            n469 = local write "X Step Size (in)"(w748) -> ()
            n470 = local write "Y Step Size (in)"(w747) -> ()
            n471 = local write "Done Mov?"(FALSE ("Done Mov?")) -> ()
          }
          frame #3 {
            n472 = property on="Move Y (in)" class="Bool (strict)"("Val(Sgnl)"=TRUE) -> (error out=w753:errorcluster)  [unwired: 2 in, 1 out]
          }
          frame #4 {
            n473 = while {
              stop <- w757 stop-if-true
              n474 = local read "Done Mov?"() -> (w757:bool)
              n475 = Wait (ms)(milliseconds to wait=u32 10 ("millisecond timer value")) -> ()  [unwired: 1 out]
            }
          }
        }
        n476 = property on="Read Position" class="Bool (strict)"("Val(Sgnl)"=TRUE) -> (error out=w729:errorcluster)  [unwired: 2 in, 1 out]
        n477 = flat-sequence {
          tunnel: w728 -> [_]
          frame #0 {
            n478 = local write "Done Mov?"(FALSE ("Done Mov?")) -> ()
            n479 = property on="Move X (in)" class="Bool (strict)"("Val(Sgnl)"=TRUE) -> ()  [unwired: 2 in, 2 out]
          }
          frame #1 {
            n480 = while {
              stop <- w736 stop-if-true
              n481 = local read "Done Mov?"() -> (w736:bool)
              n482 = Wait (ms)(milliseconds to wait=u32 10 ("millisecond timer value")) -> ()  [unwired: 1 out]
            }
          }
          frame #2 {
            n483 = local write "Done Mov?"(FALSE ("Done Mov?")) -> ()
          }
        }
      }
      frame "Move to" {
        n484 = flat-sequence {
          frame #0 {
            n485 = property on="Read Position" class="Bool (strict)"("Val(Sgnl)"=TRUE ("Value (Signaling)")) -> ()  [unwired: 2 in, 2 out]
          }
          frame #1 {
            n486 = while {
              stop <- w761 stop-if-true
              n487 = local read "Read Position"() -> (w763:bool)
              n488 = Wait (ms)(milliseconds to wait=u32 10) -> ()  [unwired: 1 out]
              n489 = Not(x=w763) -> (.not. x?=w761:bool)
            }
          }
          frame #2 {
            n490 = local read "X=T,Y=F"() -> (w765:bool)
            n491 = case shown="False" w765 {
              tunnel: [w767 w773] -> w764
              frame False {
                n492 = flat-sequence {
                  tunnel: [w771] -> w767
                  frame #0 {
                    n493 = local read "Y Pos"() -> (w769:dbl)
                    n494 = Subtract(x="Y Move", y=w769) -> (x-y=w768:dbl)
                    n495 = local write "Y Step Size (in)"(w768) -> ()
                  }
                  frame #1 {
                    n496 = property on="Move Y (in)" class="Bool (strict)"("Val(Sgnl)"=TRUE ("Value (Signaling)")) -> (error out=w771:errorcluster)  [unwired: 2 in, 1 out]
                  }
                }
              }
              frame True {
                n497 = flat-sequence {
                  tunnel: [w777] -> w773
                  frame #0 {
                    n498 = local read "X Pos"() -> (w776:dbl)
                    n499 = Subtract(x="X Move", y=w776) -> (x-y=w774:dbl)
                    n500 = local write "X Step Size (in)"(w774) -> ()
                  }
                  frame #1 {
                    n501 = property on="Move X (in)" class="Bool (strict)"("Val(Sgnl)"=TRUE ("Value (Signaling)")) -> (error out=w777:errorcluster)  [unwired: 2 in, 1 out]
                  }
                }
              }
            }
            n502 = while {
              tunnel: w764 -> [_]
              stop <- w766 stop-if-true
              n503 = local read "Done Mov?"() -> (w766:bool)
            }
          }
        }
      }
      frame "Update Vel/Acc" {
        n504 = flat-sequence {
          frame #0 {
            n505 = property on="Set Vel/Acc" class="Bool (strict)"("Val(Sgnl)"=TRUE ("Value (Signaling)")) -> ()  [unwired: 2 in, 2 out]
          }
          frame #1 {
            n506 = Wait (ms)(milliseconds to wait=u32 50) -> ()  [unwired: 1 out]
          }
        }
      }
      frame "Convert" {
        w814 = 0 ("index")
        w815 = 0 ("index")
        w812 = path "C:/Users/mnopl/OneDrive/Documents/PhiThetaScanning/GridDataScript.py" ("module path")
        n507 = local read "(X,Y)"() -> (w787:cluster{dbl, dbl}[][])
        n508 = local read "array of values"() -> (w792:dbl[][])
        n509 = Transpose 2D Array(2D array=w787) -> (transposed array=w786:cluster{dbl, dbl}[][])
        n510 = Array Size(array=w786) -> (size(s)=w826:i32[])
        n511 = Index Array(array=w826, index=0) -> (element=w818:i32)
        n512 = Index Array(array=w826, index=1) -> (element=w817:i32)
        n513 = disable-structure shown="Enabled" {
          disable-tunnel: w792 -> [w839 w840]
          disable-tunnel: [w838 w840] -> w788
          frame Disabled {
            n514 = Transpose 2D Array(2D array=w839) -> (transposed array=w838:dbl[][])
          }
          frame Enabled {
          }
        }
        n515 = Array Size(array=w788) -> (size(s)=w793:i32[])
        n516 = Index Array(array=w793, index=1) -> (element=w784:i32)
        n517 = Index Array(array=w793, index=0) -> (element=w785:i32)
        n518 = for {
          N: w785 -> [_]
          shift-right: [w842] -> w796
          shift-left: w788 -> [w843]
          tunnel: w784 -> [w841]
          i -> [w844]
          n519 = for {
            N: w841 -> [_]
            tunnel: w844 -> [w847]
            shift-right: [w845] -> w842
            shift-left: w843 -> [w848]
            i -> [w846]
            n520 = Index Array(array=w848, index (row)=w846, index (col)=w847) -> (element=w851:dbl)
            n521 = Equal?(x=-inf, y=w851) -> (x = y?=w849:bool)
            n522 = case shown="True" w849 {
              tunnel: w848 -> [w852 w857]
              tunnel: w847 -> [_ w856]
              tunnel: w846 -> [_ w855]
              tunnel: [w852 w853] -> w845
              frame False {
              }
              frame True {
                n523 = Replace Array Subset(array=w857, new element=-100.0 ("new element/subarray"), index (row)=w855, index (col)=w856) -> (w853:dbl[][])
              }
            }
          }
        }
        n524 = property on="Graph" class="IntGraph (strict)"("Active Cursor"=u32 0) -> (error out=w829:errorcluster)  [unwired: 2 in, 1 out]
        n525 = property on="Graph" class="IntGraph (strict)"(error in=w829) -> ("Cursor.Cursor Position"=w828:T1)  [unwired: 1 in, 2 out]
        n526 = for {
          N: w818 -> [_]
          tunnel: w786 -> [w862]
          tunnel: w828 -> [w860]
          tunnel: [w859] -> w790 mode=indexing
          tunnel: w817 -> [w858]
          i -> [w861]
          n527 = for {
            N: w858 -> [_]
            tunnel: w862 -> [w874]
            tunnel: w861 -> [w872]
            tunnel: w860 -> [w871]
            tunnel: [w863] -> w859 mode=indexing
            i -> [w873]
            n528 = Index Array(array=w874, index (row)=w872, index (col)=w873) -> (element=w868:cluster{dbl, dbl})
            n529 = Unbundle By Name(w871) -> ("Cursor X"=w866:dbl, "Cursor Y"=w864:dbl)
            n530 = Unbundle(w868) -> (w867:dbl, w865:dbl)
            n531 = Subtract(x=w865, y=w864) -> (x-y=w869:dbl)
            n532 = Subtract(x=w867, y=w866) -> (x-y=w870:dbl)
            n533 = Bundle(w870, w869) -> (w863:cluster{dbl, dbl})  [unwired: 1 in]
          }
        }
        n534 = Array Subset(array=w796, index (row)=w814, length (row)=w818, index (col)=w814, length (col)=w817) -> (w816:dbl[][])
        n535 = Array Size(array=w796) -> (size(s)=w822:i32[])
        n536 = Index Array(array=w822, index=1) -> (element=w820:i32)
        n537 = Index Array(array=w822, index=0) -> (element=w821:i32)
        n538 = Array Subset(array=w790, index (row)=w815, length (row)=w821, index (col)=w815, length (col)=w820) -> (w819:cluster{dbl, dbl}[][])
        n539 = node(w791, w812, "grid" ("function name"), w816, w819, w816, "Grid points") -> (w813:refnum<k35>, w806:errorcluster, w783:dbl[][])  [unwired: 4 in, 2 out]
        n540 = flat-sequence {
          tunnel: w783 -> [w835]
          tunnel: [w834] -> w789
          tunnel: w789 -> [w836]
          frame #0 {
            n541 = local write "Phi Theta Data"(w835) -> ()
            n542 = Array Max & Min(array=w835) -> (max value=w834:dbl)  [unwired: 3 out]
          }
          frame #1 {
            n543 = property on="Graph" class="IntGraph (strict)"() -> ("ZScale.Minimum"=w837:dbl)  [unwired: 2 in, 2 out]
            n544 = property on="Phi Theta Data" class="IntGraph (strict)"("ZScale.Maximum"=w836, "ZScale.Minimum"=w837) -> ()  [unwired: 2 in, 2 out]
          }
        }
        n545 = Initialize Array(0.0 ("element"), 4 ("dimension size")) -> (w808:dbl[])
        n546 = node(w813, w812, "OffsetAndMult" ("function name"), w806, w808, "Grid points") -> (w807:dbl[])  [unwired: 1 in, 4 out]
        n547 = Index Array(array=w807, index=0) -> (element=w801:dbl)
        n548 = Index Array(array=w807, index=1) -> (element=w800:dbl)
        n549 = Index Array(array=w807, index=2) -> (element=w799:dbl)
        n550 = Index Array(array=w807, index=3) -> (element=w798:dbl)
        n551 = property on="Phi Theta Data" class="IntGraph (strict)"("XScale.Multiplier"=w800, "XScale.Offset"=w801) -> ()  [unwired: 2 in, 2 out]
        n552 = property on="Phi Theta Data" class="IntGraph (strict)"("YScale.Multiplier"=w798, "YScale.Offset"=w799) -> ()  [unwired: 2 in, 2 out]
      }
      frame "Save Position" {
        n553 = flat-sequence {
          frame #0 {
            n554 = property on="Read Position" class="Bool (strict)"("Val(Sgnl)"=TRUE ("Value (Signaling)")) -> ()  [unwired: 2 in, 2 out]
          }
          frame #1 {
            n555 = while {
              stop <- w879 stop-if-true
              n556 = local read "Read Position"() -> (w880:bool)
              n557 = Wait (ms)(milliseconds to wait=u32 10) -> ()  [unwired: 1 out]
              n558 = Not(x=w880) -> (.not. x?=w879:bool)
            }
          }
          frame #2 {
            n559 = local read "X Pos"() -> (→"X Pos 1":dbl)
            n560 = local read "Y Pos"() -> (→"Y Pos 1":dbl)
          }
        }
      }
      frame "Save Image" {
        n561 = property on="Graph" class="IntGraph (strict)"("Active Cursor"=u32 0) -> (error out=w894:errorcluster)  [unwired: 2 in, 1 out]
        n562 = property on="Graph" class="IntGraph (strict)"(error in=w894, "Cursor.Visible"=FALSE) -> (error out=w888:errorcluster)  [unwired: 1 in, 1 out]
        n563 = property on="Graph" class="IntGraph (strict)"(error in=w888, "Cursor Palette Vis"=FALSE ("Cursor Legend Visible")) -> (error out=w883:errorcluster)  [unwired: 1 in, 1 out]
        n564 = invoke on="Graph" class="IntGraph (strict)" method="Get Image"(error in=w883, "image depth"=24 ("Image Depth")) -> (error out=w890:errorcluster, "image data"=w891:T2)  [unwired: 4 in, 4 out]
        n565 = call <vilib>:"Write PNG File.vi"("error in (no error)"=w890, "image data"=w891) -> ("error out"=w887:errorcluster)  [unwired: 8 in, 1 out]
        n566 = property on="Graph" class="IntGraph (strict)"(error in=w887, "Cursor.Visible"=TRUE) -> (error out=w886:errorcluster)  [unwired: 1 in, 1 out]
        n567 = property on="Graph" class="IntGraph (strict)"(error in=w886, "Cursor Palette Vis"=TRUE ("Cursor.Visible")) -> ()  [unwired: 1 in, 2 out]
      }
      frame "Save Data" {
        w909 = 0 ("index")
        w921 = 0
        n568 = local read "(X,Y)"() -> (w905:cluster{dbl, dbl}[][])
        n569 = Array Size(array=w905) -> (size(s)=w900:i32[])
        n570 = Index Array(array=w900, index=0) -> (element=w903:i32)
        n571 = Index Array(array=w900, index=1) -> (element=w902:i32)
        n572 = property on="Graph" class="IntGraph (strict)"("Active Cursor"=u32 0) -> (error out=w899:errorcluster)  [unwired: 2 in, 1 out]
        n573 = property on="Graph" class="IntGraph (strict)"(error in=w899) -> ("Cursor.Cursor Position"=w906:T1)  [unwired: 1 in, 2 out]
        n574 = for {
          N: w903 -> [_]
          tunnel: w905 -> [w933]
          tunnel: w906 -> [w931]
          tunnel: [w930] -> w907 mode=indexing
          tunnel: w902 -> [w929]
          i -> [w932]
          n575 = for {
            N: w929 -> [_]
            tunnel: w933 -> [w945]
            tunnel: w932 -> [w943]
            tunnel: w931 -> [w942]
            tunnel: [w934] -> w930 mode=indexing
            i -> [w944]
            n576 = Index Array(array=w945, index (row)=w943, index (col)=w944) -> (element=w939:cluster{dbl, dbl})
            n577 = Unbundle By Name(w942) -> ("Cursor X"=w937:dbl, "Cursor Y"=w935:dbl)
            n578 = Unbundle(w939) -> (w938:dbl, w936:dbl)
            n579 = Subtract(x=w936, y=w935) -> (x-y=w940:dbl)
            n580 = Subtract(x=w938, y=w937) -> (x-y=w941:dbl)
            n581 = Bundle(w941, w940) -> (w934:cluster{dbl, dbl})  [unwired: 1 in]
          }
        }
        n582 = local read "array of values"() -> (w922:dbl[][])
        n583 = Array Size(array=w907) -> (size(s)=w918:i32[])
        n584 = Index Array(array=w918, index=0) -> (element=w919:i32)
        n585 = Index Array(array=w918, index=1) -> (element=w916:i32)
        n586 = Array Size(array=w922) -> (size(s)=w914:i32[])
        n587 = Array Subset(array=w922, index (row)=w921, length (row)=w919, index (col)=w921, length (col)=w916) -> (w915:dbl[][])
        n588 = Index Array(array=w914, index=0) -> (element=w910:i32)
        n589 = Index Array(array=w914, index=1) -> (element=w911:i32)
        n590 = Array Subset(array=w907, index (row)=w909, length (row)=w910, index (col)=w909, length (col)=w911) -> (w908:cluster{dbl, dbl}[][])
        n591 = node(w928, path "C:/Users/mnopl/OneDrive/Documents/PhiThetaScanning/SaveDataToTextFiles.py" ("module path"), "savedata" ("function name"), w915, w908, w915) -> (→"return value":dbl[][])  [unwired: 3 in, 4 out]
      }
      frame "Save Phi/Theta" {
        n592 = property on="Phi Theta Data" class="IntGraph (strict)"("Active Cursor"=u32 0) -> (error out=w956:errorcluster)  [unwired: 2 in, 1 out]
        n593 = property on="Phi Theta Data" class="IntGraph (strict)"(error in=w956, "Cursor.Visible"=FALSE) -> (error out=w954:errorcluster)  [unwired: 1 in, 1 out]
        n594 = property on="Phi Theta Data" class="IntGraph (strict)"(error in=w954, "Cursor Palette Vis"=FALSE ("Cursor Legend Visible")) -> (error out=w952:errorcluster)  [unwired: 1 in, 1 out]
        n595 = invoke on="Phi Theta Data" class="IntGraph (strict)" method="Get Image"(error in=w952, "image depth"=24 ("Image Depth")) -> ("image data"=w951:T2)  [unwired: 4 in, 5 out]
        n596 = call <vilib>:"Write PNG File.vi"("image data"=w951) -> ("error out"=w950:errorcluster)  [unwired: 9 in, 1 out]
        n597 = property on="Phi Theta Data" class="IntGraph (strict)"(error in=w950, "Cursor.Visible"=TRUE) -> (error out=w949:errorcluster)  [unwired: 1 in, 1 out]
        n598 = property on="Phi Theta Data" class="IntGraph (strict)"(error in=w949, "Cursor Palette Vis"=TRUE ("Cursor Legend Visible")) -> ()  [unwired: 1 in, 2 out]
      }
      frame "Save Line graph" {
        n599 = property on="Line Scan" class="WFGraph (strict)"("Active Cursor"=u32 0) -> (error out=w966:errorcluster)  [unwired: 2 in, 1 out]
        n600 = property on="Line Scan" class="WFGraph (strict)"(error in=w966, "Cursor.Visible"=FALSE) -> (error out=w967:errorcluster)  [unwired: 1 in, 1 out]
        n601 = property on="Line Scan" class="WFGraph (strict)"(error in=w967, "Cursor Palette Vis"=FALSE ("Cursor Legend Visible")) -> (error out=w968:errorcluster)  [unwired: 1 in, 1 out]
        n602 = invoke on="Line Scan" class="WFGraph (strict)" method="Get Image"(error in=w968, "image depth"=24 ("Image Depth")) -> (error out=w970:errorcluster, "image data"=w969:T2)  [unwired: 4 in, 4 out]
        n603 = call <vilib>:"Write PNG File.vi"("error in (no error)"=w970, "image data"=w969) -> ("error out"=w971:errorcluster)  [unwired: 8 in, 1 out]
        n604 = property on="Line Scan" class="WFGraph (strict)"(error in=w971, "Cursor.Visible"=TRUE) -> (error out=w972:errorcluster)  [unwired: 1 in, 1 out]
        n605 = property on="Line Scan" class="WFGraph (strict)"(error in=w972, "Cursor Palette Vis"=TRUE ("Cursor Legend Visible")) -> ()  [unwired: 1 in, 2 out]
      }
      frame "Stop" {
      }
    }
  }
  n606 = while {
    shift-right: [w980] -> _
    shift-left: "Idle" -> [w981]
    tunnel: [w978] -> w8
    tunnel: w2 -> [w978]
    tunnel: [w977] -> w7
    tunnel: w1 -> [w977]
    stop <- w979 stop-if-true
    n607 = case shown="\"Idle\", Default" w981 {
      tunnel: [w983 "Wait" "Wait" "Idle" "Idle" "Idle"] -> w980
      tunnel: [FALSE TRUE FALSE FALSE FALSE FALSE] -> w979
      tunnel: w978 -> [_ _ w1000 w1013 _ w1029]
      tunnel: w977 -> [_ _ w999 w1014 _ w1030]
      frame "Idle", Default {
        # "Might not be necesarry"
        n608 = flat-sequence {
          frame #0 {
            w984 = FALSE
            n609 = local write "Read Position"(w984) -> ()
            n610 = local write "Moving?"(w984) -> ()
            n611 = local write "Set Vel/Acc"(w984) -> ()
          }
        }
        n612 = event shown="[3] \"Set Vel/Acc\": Value Change" {
          selector: _ -> [_ _ _ _ _]
          dyn-events: _ -> [_ _ _ _ _]
          timeout: _ -> [_ _ _ _ _]
          tunnel: ["Idle" "Moving" "Read Position" "Set Vel/Acc" "Stop"] -> w983
          event Timeout {
            n613 = event-data() -> ()  [unwired: 1 in, 3 out]
          }
          event "Moving?": Value Change {
            n614 = event-data() -> ()  [unwired: 1 in, 6 out]
          }
          event "Read Position": Value Change {
            n615 = event-data() -> ()  [unwired: 1 in, 6 out]
          }
          event "Set Vel/Acc": Value Change {
            n616 = event-data() -> ()  [unwired: 1 in, 6 out]
          }
          event "Stop": Value Change {
            n617 = event-data() -> ()  [unwired: 1 in, 6 out]
          }
        }
      }
      frame "Stop" {
      }
      frame "Moving" {
        n618 = case shown="True" "X=T,Y=F" {
          tunnel: w1000 -> [_ w1007]
          tunnel: w999 -> [w1005 _]
          tunnel: [w1005 w1007] -> w992
          tunnel: [w1004 w1006] -> w996
          frame False {
            n619 = local read "Y Step Size (in)"() -> (w1004:dbl)
          }
          frame True {
            n620 = local read "X Step Size (in)"() -> (w1006:dbl)
          }
        }
        n621 = invoke class="KCubeStepper" method="SetMoveRelativeDistance"(reference=w992, "distance"=w996) -> (reference out=w998:refnum<k24>, error out=w997:errorcluster)  [unwired: 2 in, 2 out]
        n622 = invoke class="KCubeStepper" method="MoveRelative"(reference=w998, error in=w997, "waitTimeout"=0) -> (error out=w995:errorcluster)  [unwired: 1 in, 3 out]
        n623 = flat-sequence {
          tunnel: w995 -> [_]
          frame #0 {
            n624 = Tick Count (ms)() -> (millisecond timer value=→"Time":u32)
          }
        }
      }
      frame "Set Vel/Acc" {
        n625 = local read "Velocity"() -> (w1011:dbl)
        n626 = local read "Acceleration"() -> (w1010:dbl)
        n627 = invoke class="KCubeStepper" method="SetVelocityParams"(reference=w1014, "maxVelocity"=w1011, "acceleration"=w1010) -> (error out=w1012:errorcluster)  [unwired: 2 in, 4 out]
        n628 = invoke class="KCubeStepper" method="SetVelocityParams"(reference=w1013, error in=w1012, "maxVelocity"=w1011, "acceleration"=w1010) -> ()  [unwired: 1 in, 5 out]
      }
      frame "Wait" {
        n629 = while {
          tunnel: [FALSE] -> w1015
          stop <- w1019 stop-if-true
          n630 = local read "Time"() -> (w1024:i32)
          n631 = Tick Count (ms)() -> (millisecond timer value=w1023:u32)
          n632 = Subtract(x=w1023, y=w1024) -> (x-y=w1021:u32)
          n633 = Greater Or Equal?(x=w1021, y="Time to wait") -> (x >= y?=w1019:bool)
          "Done Mov?" <- w1019
        }
        n634 = flat-sequence {
          tunnel: w1015 -> [w1018]
          frame #0 {
            n635 = local write "Move Y (in)"(w1018) -> ()
            n636 = local write "Move X (in)"(w1018) -> ()
          }
        }
      }
      frame "Read Position" {
        n637 = invoke class="KCubeStepper" method="GetPositionCounter"(reference=w1029) -> ("GetPositionCounter"=w1027:i32)  [unwired: 2 in, 2 out]
        n638 = invoke class="KCubeStepper" method="GetPositionCounter"(reference=w1030) -> ("GetPositionCounter"=w1032:i32)  [unwired: 2 in, 2 out]
        n639 = Divide(x=w1027, y=2184560) -> (x/y=w1028:dbl)
        n640 = Divide(x=w1032, y=2184560) -> (x/y=w1031:dbl)
        n641 = flat-sequence {
          tunnel: w1031 -> [w1036]
          tunnel: w1028 -> [w1037]
          frame #0 {
            n642 = local write "X Pos"(w1037) -> ()
            n643 = local write "Y Pos"(w1036) -> ()
            n644 = Wait (ms)(milliseconds to wait=u32 150) -> ()  [unwired: 1 out]
            n645 = local write "Read Position"(FALSE) -> ()
          }
        }
      }
    }
  }
  n646 = while {
    tunnel: w5 -> [_]
    shift-right: [w1040] -> _
    shift-left: "Idle" -> [w1041]
    stop <- w1039 stop-if-true
    n647 = case shown="\"Moving\"" w1041 {
      tunnel: [w1043 "Stop" "Idle"] -> w1040
      tunnel: [FALSE TRUE FALSE] -> w1039
      frame "Idle", Default {
        n648 = flat-sequence {
          frame #0 {
            w1044 = FALSE
            n649 = local write "Move X (in)"(w1044) -> ()
            n650 = local write "Move Y (in)"(w1044) -> ()
            n651 = local write "Take Single Measurement"(w1044) -> ()
            n652 = local write "Moving?"(w1044) -> ()
            n653 = local write "Move X"(w1044) -> ()
            n654 = local write "Move Y"(w1044) -> ()
          }
        }
        n655 = event shown="[5] \"Move Y (in)\": Value Change" {
          selector: _ -> [_ _ _ _ _ _ _]
          dyn-events: _ -> [_ _ _ _ _ _ _]
          timeout: _ -> [_ _ _ _ w1052 _ _]
          tunnel: ["Wait" "Stop" "Moving" "Moving" "Moving" "Moving" "Idle"] -> w1043
          tunnel: [_ _ _ _ w1052 _ _] -> _
          event Timeout {
            n656 = event-data() -> ()  [unwired: 1 in, 3 out]
          }
          event "Stop": Value Change {
            n657 = event-data() -> ()  [unwired: 1 in, 6 out]
          }
          event "Move X (in)": Value Change {
            n658 = event-data() -> ()  [unwired: 1 in, 6 out]
            n659 = local write "X=T,Y=F"(TRUE) -> ()
          }
          event "Move X": Value Change {
            n660 = event-data() -> ()  [unwired: 1 in, 6 out]
            n661 = local write "X Step Size (in)"("X Step Size") -> ()
            n662 = local write "X=T,Y=F"(TRUE ("X=T,Y=F")) -> ()
          }
          event "Move Y": Value Change {
            n663 = event-data() -> ()  [unwired: 1 in, 6 out]
            n664 = local write "X=T,Y=F"(FALSE ("X=T,Y=F")) -> ()
            n665 = local write "Y Step Size (in)"("Y Step Size") -> ()
          }
          event "Move Y (in)": Value Change {
            n666 = event-data() -> ()  [unwired: 1 in, 6 out]
            n667 = local write "X=T,Y=F"(FALSE) -> ()
          }
          event "Take Single Measurement": Value Change {
            n668 = event-data() -> ()  [unwired: 1 in, 6 out]
          }
        }
      }
      frame "Stop" {
      }
      frame "Moving" {
        n669 = local read "X=T,Y=F"() -> (w1072:bool)
        n670 = case shown="False" w1072 {
          tunnel: [w1103 w1105] -> w1071
          frame False {
            n671 = Absolute Value(x="Y Step Size (in)") -> (abs(x)=w1103:dbl)
          }
          frame True {
            n672 = Absolute Value(x="X Step Size (in)") -> (abs(x)=w1105:dbl)
          }
        }
        n673 = local read "Velocity"() -> (w1064:dbl)
        n674 = Divide(x=w1064, y=1.0) -> (x/y=w1068:dbl)
        n675 = Divide(x=w1064, y="Acceleration") -> (x/y=w1063:dbl)
        n676 = Multiply(x=w1063, y=1000.0) -> (x*y=w1061:dbl)
        n677 = disable-structure shown="Enabled" {
          disable-tunnel: w1071 -> [w1083 w1094]
          disable-tunnel: [w1078 w1086] -> w1069
          disable-tunnel: w1068 -> [w1079 w1084]
          disable-tunnel: w1061 -> [w1076 _]
          frame Enabled {
            n678 = Absolute Value(x=w1083) -> (abs(x)=w1081:dbl)
            n679 = Divide(x=w1081, y=w1079) -> (x/y=w1082:dbl)
            n680 = Multiply(x=w1082, y=1000.0) -> (x*y=w1077:dbl)
            n681 = Add(x=w1076, y=50.0) -> ()  [unwired: 1 out]
            n682 = Add(x=250.0, y=w1077) -> (x+y=w1078:dbl)
          }
          frame Disabled {
            w1090 = 10.0 ("y")
            # "Acceleration"
            n683 = Multiply(x=w1094, y=2.0) -> (x*y=w1092:dbl)
            n684 = Square(x=w1084) -> (x^2=w1095:dbl)
            n685 = Multiply(x=w1092, y=w1090) -> (x*y=w1093:dbl)
            n686 = Add(x=w1095, y=w1093) -> (x+y=w1096:dbl)
            n687 = Negate(x=w1084) -> (-x=w1099:dbl)
            n688 = Square Root(x=w1096) -> (sqrt(x)=w1098:dbl)
            n689 = Add(x=w1099, y=w1098) -> (x+y=w1097:dbl)
            n690 = Divide(x=w1097, y=w1090) -> (x/y=w1089:dbl)
            n691 = Multiply(x=w1089, y=1000.0) -> (x*y=w1087:dbl)
            n692 = Add(x=w1087, y=0.0) -> (x+y=w1086:dbl)
          }
        }
        n693 = flat-sequence {
          tunnel: w1069 -> [w1101]
          tunnel: [w1100] -> w1066
          tunnel: w1066 -> [_]
          frame #0 {
            n694 = Round Toward +Infinity(x=w1101) -> (ceil(x): smallest int >= x=w1100:dbl)
            n695 = local write "Time to wait"(w1100) -> ()
            n696 = property on="Moving?" class="Bool (strict)"("Val(Sgnl)"=TRUE) -> ()  [unwired: 2 in, 2 out]
          }
          frame #1 {
          }
        }
      }
    }
  }
  n697 = flat-sequence {
    tunnel: w8 -> [w1109]
    tunnel: w7 -> [w1108]
    frame #0 {
      n698 = invoke class="KCubeStepper" method="Disconnect"(reference=w1109) -> ()  [unwired: 2 in, 3 out]
      n699 = invoke class="KCubeStepper" method="Disconnect"(reference=w1108) -> ()  [unwired: 2 in, 3 out]
      n700 = local write "Stop"(FALSE ("Stop")) -> ()
    }
  }
  n701 = Close Python Session(session in=w3) -> ()  [unwired: 1 in, 1 out]
